vi "FlexDDS-NG_USB_ExampleJTedit.vi"() -> ()   [LabVIEW 2016]
uses:
  <vilib>/Utility/xml.llb/Read From XML File(string).vi
  <vilib>/Utility/xml.llb/Write to XML File(string).vi
panel:
  in  "Interactive on/off":T1(ring)
  out "return count":u32=6435
  in  "Store data":enum32{"Save settings", "Don't save settings"}(tab)=enum."Don't save settings"
  in  "XML File Path WRITE":path=path "U:/Dokumente/Bachelorarbeit/Labview/FlexDDS-NG/conf/settings_s_curve_up_down.xml"
  in  "Data source":T2(tab)=enum."Generate data with function"
  in  "XML File Path READ":path=path "U:/Dokumente/Bachelorarbeit/Labview/FlexDDS-NG/conf/settings_4consecutive_falling.xml"
  in  "Select curve form":enum32{"S curve", "Exp curve"}(tab)
  in  "s curve parameters":cluster{"k":dbl}={"k"=10.0}
  in  "exp curve parameters":cluster{"k":dbl}={"k"=5.0}
  in  "parameters non-constant channel":T3={"Number of steps"=40, "time [ms]"=10000.0, "start frequency [Hz]"=80000000.0, "end frequency [Hz]"=82000000.0}
  in  "constant frequency":dbl=80000000.0 format="%#_13g"
  in  "Constant Channel":T4(ring)
  in  "CFR2 bits":T5={"Enable ASF from STP (F)"=FALSE, "Digital ramp enable (F)"=TRUE, "Digital ramp no-dwell high (F)"=FALSE, "Digital ramp no-dwell low (F)"=FALSE, "Matched latency enable (T)"=TRUE, "Parallel data port enable (F)"=FALSE}
  in  "CFR1 bits":T6={"RAM enable (F)"=FALSE, "Manual OSK external control (F)"=FALSE, "Inverse sinc filter enable (T)"=TRUE, "DDS sine (/cosine) output (F)"=FALSE, "Load LRR at I/O update (F)"=FALSE, "Autoclear digital ramp accumulator (F)"=TRUE, "Autoclear phase accumulator (F)"=FALSE, "Clear digital ramp accumulator (F)"=FALSE, "Clear phase accumulator (F)"=FALSE, "Load ARR at I/O update (F)"=FALSE, "OSK enable (F)"=FALSE, "Select Auto OSK (F)"=FALSE}
  in  "Trigger before sequence of sweeps":T7(ring)
  out "appended instruction string 2":string="dds reset\rdcp spi:CFR1=0x404000\rdcp spi:CFR2=0x80080\rdcp 0 spi:STP0=0x3FFF0000028F5C29\rdcp 1 spi:STP0=0x3FFF0000028F5C29\rdcp 0 spi:DRL=0x147C0118147BC1DB\rdcp 0 spi:DRSS=0xFFFFFFFF00000003\rdcp 0 spi:DRR=0x2D3E\rdcp 0 update:u-d\rdcp 0 update:+d\rdcp 1 spi:DRL=0x147AE148147AE148\rdcp 1 spi:DRSS=0xFFFFFFFF00000000\rdcp 1 spi:DRR=0xFFFF\rdcp 1 update:u-d\rdcp 1 update:+d\rdcp wait:1h:\rdcp wait::DROVER\rdcp 0 spi:DRL=0x147C51F1147C0118\rdcp 0 spi:DRSS=0xFFFFFFFF00000004\rdcp 0 spi:DRR=0x2F2F\rdcp 0 update:u-d\rdcp 0 update:+d\rdcp wait:1h:\rdcp wait::DROVER\rdcp 0 spi:DRL=0x147CB92D147C51F1\rdcp 0 spi:DRSS=0xFFFFFFFF00000017\rdcp 0 spi:DRR=0xD478\rdcp 0 update:u-d\rdcp 0 update:+d\rdcp wait:1h:\rdcp wait::DROVER\rdcp 0 spi:DRL=0x147D3CCC147CB92D\rdcp 0 spi:DRSS=0xFFFFFFFF00000009\rdcp 0 spi:DRR=0x4136\rdcp 0 update:u-d\rdcp 0 update:+d\rdcp wait:1h:\rdcp wait::DROVER\rdcp 0 spi:DRL=0x147DE446147D3CCC\rdcp 0 spi:DRSS=0xFFFFFFFF0000000D\rdcp 0 spi:DRR=0x4A07\rdcp 0 update:u-d\rdcp 0 update:+d\rdcp wait:1h:\rdcp wait::DROVER\rdcp 0 spi:DRL=0x147EB8D6147DE446\rdcp 0 spi:DRSS=0xFFFFFFFF0000002B\rdcp 0 spi:DRR=0xC0EC\rdcp 0 update:u-d\rdcp 0 update:+d\rdcp wait:1h:\rdcp wait::DROVER\rdcp 0 spi:DRL=0x147FC5C3147EB8D6\rdcp 0 spi:DRSS=0xFFFFFFFF00000006\rdcp 0 spi:DRR=0x1547\rdcp 0 update:u-d\rdcp 0 update:+d\rdcp wait:1h:\rdcp wait::DROVER\rdcp 0 spi:DRL=0x148118A1147FC5C3\rdcp 0 spi:DRSS=0xFFFFFFFF0000001C\rdcp 0 spi:DRR=0x4ECD\rdcp 0 update:u-d\rdcp 0 update:+d\rdcp wait:1h:\rdcp wait::DROVER\rdcp 0 spi:DRL=0x1482C174148118A1\rdcp 0 spi:DRSS=0xFFFFFFFF00000049\rdcp 0 spi:DRR=0xA3E0\rdcp 0 update:u-d\rdcp 0 update:+d\rdcp wait:1h:\rdcp wait::DROVER\rdcp 0 spi:DRL=0x1484D2A81482C174\rdcp 0 spi:DRSS=0xFFFFFFFF00000003\rdcp 0 spi:DRR=0x568\rdcp 0 update:u-d\rdcp 0 update:+d\rdcp wait:1h:\rdcp wait::DROVER\rdcp 0 spi:DRL=0x148760AD1484D2A8\rdcp 0 spi:DRSS=0xFFFFFFFF0000008C\rdcp 0 spi:DRR=0xCC25\rdcp 0 update:u-d\rdcp 0 update:+d\rdcp wait:1h:\rdcp wait::DROVER\rdcp 0 spi:DRL=0x148A8111148760AD\rdcp 0 spi:DRSS=0xFFFFFFFF00000049\rdcp 0 spi:DRR=0x56FB\rdcp 0 update:u-d\rdcp 0 update:+d\rdcp wait:1h:\rdcp wait::DROVER\rdcp 0 spi:DRL=0x148E48EB148A8111\rdcp 0 spi:DRSS=0xFFFFFFFF00000004\rdcp 0 spi:DRR=0x3F1\rdcp 0 update:u-d\rdcp 0 update:+d\rdcp wait:1h:\rdcp wait::DROVER\rdcp 0 spi:DRL=0x1492CA77148E48EB\rdcp 0 spi:DRSS=0xFFFFFFFF000000A0\rdcp 0 spi:DRR=0x8447\rdcp 0 update:u-d\rdcp 0 update:+d\rdcp wait:1h:\rdcp wait::DROVER\rdcp 0 spi:DRL=0x149811DB1492CA77\rdcp 0 spi:DRSS=0xFFFFFFFF000000D0\rdcp 0 spi:DRR=0x92C9\rdcp 0 update:u-d\rdcp 0 update:+d\rdcp wait:1h:\rdcp wait::DROVER\rdcp 0 spi:DRL=0x149E2175149811DB\rdcp 0 spi:DRSS=0xFFFFFFFF00000100\rdcp 0 spi:DRR=0x9D59\rdcp 0 update:u-d\rdcp 0 update:+d\rdcp wait:1h:\rdcp wait::DROVER\rdcp 0 spi:DRL=0x14A4EE42149E2175\rdcp 0 spi:DRSS=0xFFFFFFFF000000C7\rdcp 0 spi:DRR=0x6D05\rdcp 0 update:u-d\rdcp 0 update:+d\rdcp wait:1h:\rdcp wait::DROVER\rdcp 0 spi:DRL=0x14AC5D7114A4EE42\rdcp 0 spi:DRSS=0xFFFFFFFF00000019\rdcp 0 spi:DRR=0xC87\rdcp 0 update:u-d\rdcp 0 update:+d\rdcp wait:1h:\rdcp wait::DROVER\rdcp 0 spi:DRL=0x14B4443314AC5D71\rdcp 0 spi:DRSS=0xFFFFFFFF00000021\rdcp 0 spi:DRR=0xF8F\rdcp 0 update:u-d\rdcp 0 update:+d\rdcp wait:1h:\rdcp wait::DROVER\rdcp 0 spi:DRL=0x14BC6A7F14B44433\rdcp 0 spi:DRSS=0xFFFFFFFF0000014D\rdcp 0 spi:DRR=0x9838\rdcp 0 update:u-d\rdcp 0 update:+d\rdcp wait:1h:\rdcp wait::DROVER\rdcp 0 spi:DRL=0x14C490CB14BC6A7F\rdcp 0 spi:DRSS=0xFFFFFFFF0000014D\rdcp 0 spi:DRR=0x9838\rdcp 0 update:u-d\rdcp 0 update:+d\rdcp wait:1h:\rdcp wait::DROVER\rdcp 0 spi:DRL=0x14CC778D14C490CB\rdcp 0 spi:DRSS=0xFFFFFFFF00000021\rdcp 0 spi:DRR=0xF8F\rdcp 0 update:u-d\rdcp 0 update:+d\rdcp wait:1h:\rdcp wait::DROVER\rdcp 0 spi:DRL=0x14D3E6BC14CC778D\rdcp 0 spi:DRSS=0xFFFFFFFF00000019\rdcp 0 spi:DRR=0xC87\rdcp 0 update:u-d\rdcp 0 update:+d\rdcp wait:1h:\rdcp wait::DROVER\rdcp 0 spi:DRL=0x14DAB38914D3E6BC\rdcp 0 spi:DRSS=0xFFFFFFFF000000C7\rdcp 0 spi:DRR=0x6D05\rdcp 0 update:u-d\rdcp 0 update:+d\rdcp wait:1h:\rdcp wait::DROVER\rdcp 0 spi:DRL=0x14E0C32314DAB389\rdcp 0 spi:DRSS=0xFFFFFFFF00000100\rdcp 0 spi:DRR=0x9D59\rdcp 0 update:u-d\rdcp 0 update:+d\rdcp wait:1h:\rdcp wait::DROVER\rdcp 0 spi:DRL=0x14E60A8714E0C323\rdcp 0 spi:DRSS=0xFFFFFFFF000000D0\rdcp 0 spi:DRR=0x92C9\rdcp 0 update:u-d\rdcp 0 update:+d\rdcp wait:1h:\rdcp wait::DROVER\rdcp 0 spi:DRL=0x14EA8C1314E60A87\rdcp 0 spi:DRSS=0xFFFFFFFF000000A0\rdcp 0 spi:DRR=0x8447\rdcp 0 update:u-d\rdcp 0 update:+d\rdcp wait:1h:\rdcp wait::DROVER\rdcp 0 spi:DRL=0x14EE53ED14EA8C13\rdcp 0 spi:DRSS=0xFFFFFFFF00000004\rdcp 0 spi:DRR=0x3F1\rdcp 0 update:u-d\rdcp 0 update:+d\rdcp wait:1h:\rdcp wait::DROVER\rdcp 0 spi:DRL=0x14F1745114EE53ED\rdcp 0 spi:DRSS=0xFFFFFFFF00000049\rdcp 0 spi:DRR=0x56FB\rdcp 0 update:u-d\rdcp 0 update:+d\rdcp wait:1h:\rdcp wait::DROVER\rdcp 0 spi:DRL=0x14F4025514F17451\rdcp 0 spi:DRSS=0xFFFFFFFF0000008C\rdcp 0 spi:DRR=0xCC25\rdcp 0 update:u-d\rdcp 0 update:+d\rdcp wait:1h:\rdcp wait::DROVER\rdcp 0 spi:DRL=0x14F6138A14F40255\rdcp 0 spi:DRSS=0xFFFFFFFF00000003\rdcp 0 spi:DRR=0x568\rdcp 0 update:u-d\rdcp 0 update:+d\rdcp wait:1h:\rdcp wait::DROVER\rdcp 0 spi:DRL=0x14F7BC5D14F6138A\rdcp 0 spi:DRSS=0xFFFFFFFF00000049\rdcp 0 spi:DRR=0xA3E0\rdcp 0 update:u-d\rdcp 0 update:+d\rdcp wait:1h:\rdcp wait::DROVER\rdcp 0 spi:DRL=0x14F90F3B14F7BC5D\rdcp 0 spi:DRSS=0xFFFFFFFF0000001C\rdcp 0 spi:DRR=0x4ECD\rdcp 0 update:u-d\rdcp 0 update:+d\rdcp wait:1h:\rdcp wait::DROVER\rdcp 0 spi:DRL=0x14FA1C2814F90F3B\rdcp 0 spi:DRSS=0xFFFFFFFF00000006\rdcp 0 spi:DRR=0x1547\rdcp 0 update:u-d\rdcp 0 update:+d\rdcp wait:1h:\rdcp wait::DROVER\rdcp 0 spi:DRL=0x14FAF0B814FA1C28\rdcp 0 spi:DRSS=0xFFFFFFFF0000002B\rdcp 0 spi:DRR=0xC0EC\rdcp 0 update:u-d\rdcp 0 update:+d\rdcp wait:1h:\rdcp wait::DROVER\rdcp 0 spi:DRL=0x14FB983214FAF0B8\rdcp 0 spi:DRSS=0xFFFFFFFF0000000D\rdcp 0 spi:DRR=0x4A07\rdcp 0 update:u-d\rdcp 0 update:+d\rdcp wait:1h:\rdcp wait::DROVER\rdcp 0 spi:DRL=0x14FC1BD114FB9832\rdcp 0 spi:DRSS=0xFFFFFFFF00000009\rdcp 0 spi:DRR=0x4136\rdcp 0 update:u-d\rdcp 0 update:+d\rdcp wait:1h:\rdcp wait::DROVER\rdcp 0 spi:DRL=0x14FC830D14FC1BD1\rdcp 0 spi:DRSS=0xFFFFFFFF00000017\rdcp 0 spi:DRR=0xD478\rdcp 0 update:u-d\rdcp 0 update:+d\rdcp wait:1h:\rdcp wait::DROVER\rdcp 0 spi:DRL=0x14FCD3E614FC830D\rdcp 0 spi:DRSS=0xFFFFFFFF00000004\rdcp 0 spi:DRR=0x2F2F\rdcp 0 update:u-d\rdcp 0 update:+d\rdcp wait:1h:\rdcp wait::DROVER\rdcp 0 spi:DRL=0x14FD132314FCD3E6\rdcp 0 spi:DRSS=0xFFFFFFFF00000003\rdcp 0 spi:DRR=0x2D3E\rdcp 0 update:u-d\rdcp 0 update:+d\rdcp wait:1h:\rdcp wait::DROVER\rdcp 0 spi:DRL=0x14FD448E14FD1323\rdcp 0 spi:DRSS=0xFFFFFFFF00000002\rdcp 0 spi:DRR=0x2699\rdcp 0 update:u-d\rdcp 0 update:+d\rdcp wait:1h:\rdcp wait::DROVER\rdcp start\r"
  out "frequency-time plot":T8(graph)=[{[{"total time[ms]"=0.0, "f1 [Hz] CH0"=80013385.70184857}, {"total time[ms]"=250.0, "f1 [Hz] CH0"=80017154.97082743}, {"total time[ms]"=250.0, "f1 [Hz] CH0"=80017154.97082743}, {"total time[ms]"=500.0, "f1 [Hz] CH0"=80021973.8852612}, {"total time[ms]"=500.0, "f1 [Hz] CH0"=80021973.8852612}, {"total time[ms]"=750.0, "f1 [Hz] CH0"=80028127.2540865}, {"total time[ms]"=750.0, "f1 [Hz] CH0"=80028127.2540865}, {"total time[ms]"=1000.0, "f1 [Hz] CH0"=80035972.41992418}, {"total time[ms]"=1000.0, "f1 [Hz] CH0"=80035972.41992418}, {"total time[ms]"=1250.0, "f1 [Hz] CH0"=80045954.73982005}, {"total time[ms]"=1250.0, "f1 [Hz] CH0"=80045954.73982005}, {"total time[ms]"=1500.0, "f1 [Hz] CH0"=80058624.46150272}, {"total time[ms]"=1500.0, "f1 [Hz] CH0"=80058624.46150272}, {"total time[ms]"=1750.0, "f1 [Hz] CH0"=80074653.77468826}, {"total time[ms]"=1750.0, "f1 [Hz] CH0"=80074653.77468826}, {"total time[ms]"=2000.0, "f1 [Hz] CH0"=80094851.74635513}, {"total time[ms]"=2000.0, "f1 [Hz] CH0"=80094851.74635513}, {"total time[ms]"=2250.0, "f1 [Hz] CH0"=80120173.30034801}, {"total time[ms]"=2250.0, "f1 [Hz] CH0"=80120173.30034801}, {"total time[ms]"=2500.0, "f1 [Hz] CH0"=80151716.36004248}, {"total time[ms]"=2500.0, "f1 [Hz] CH0"=80151716.36004248}, {"total time[ms]"=2750.0, "f1 [Hz] CH0"=80190698.92979822}, {"total time[ms]"=2750.0, "f1 [Hz] CH0"=80190698.92979822}, {"total time[ms]"=3000.0, "f1 [Hz] CH0"=80238405.84404424}, {"total time[ms]"=3000.0, "f1 [Hz] CH0"=80238405.84404424}, {"total time[ms]"=3250.0, "f1 [Hz] CH0"=80296094.39606337}, {"total time[ms]"=3250.0, "f1 [Hz] CH0"=80296094.39606337}, {"total time[ms]"=3500.0, "f1 [Hz] CH0"=80364851.04761271}, {"total time[ms]"=3500.0, "f1 [Hz] CH0"=80364851.04761271}, {"total time[ms]"=3750.0, "f1 [Hz] CH0"=80445400.27765062}, {"total time[ms]"=3750.0, "f1 [Hz] CH0"=80445400.27765062}, {"total time[ms]"=4000.0, "f1 [Hz] CH0"=80537882.84273998}, {"total time[ms]"=4000.0, "f1 [Hz] CH0"=80537882.84273998}, {"total time[ms]"=4250.0, "f1 [Hz] CH0"=80641642.60164921}, {"total time[ms]"=4250.0, "f1 [Hz] CH0"=80641642.60164921}, {"total time[ms]"=4500.0, "f1 [Hz] CH0"=80755081.3375963}, {"total time[ms]"=4500.0, "f1 [Hz] CH0"=80755081.3375963}, {"total time[ms]"=4750.0, "f1 [Hz] CH0"=80875646.9982284}, {"total time[ms]"=4750.0, "f1 [Hz] CH0"=80875646.9982284}, {"total time[ms]"=5000.0, "f1 [Hz] CH0"=81000000.0}, {"total time[ms]"=5000.0, "f1 [Hz] CH0"=81000000.0}, {"total time[ms]"=5250.0, "f1 [Hz] CH0"=81124353.0017716}, {"total time[ms]"=5250.0, "f1 [Hz] CH0"=81124353.0017716}, {"total time[ms]"=5500.0, "f1 [Hz] CH0"=81244918.6624037}, {"total time[ms]"=5500.0, "f1 [Hz] CH0"=81244918.6624037}, {"total time[ms]"=5750.0, "f1 [Hz] CH0"=81358357.39835079}, {"total time[ms]"=5750.0, "f1 [Hz] CH0"=81358357.39835079}, {"total time[ms]"=6000.0, "f1 [Hz] CH0"=81462117.15726002}, {"total time[ms]"=6000.0, "f1 [Hz] CH0"=81462117.15726002}, {"total time[ms]"=6250.0, "f1 [Hz] CH0"=81554599.72234938}, {"total time[ms]"=6250.0, "f1 [Hz] CH0"=81554599.72234938}, {"total time[ms]"=6500.0, "f1 [Hz] CH0"=81635148.95238729}, {"total time[ms]"=6500.0, "f1 [Hz] CH0"=81635148.95238729}, {"total time[ms]"=6750.0, "f1 [Hz] CH0"=81703905.60393663}, {"total time[ms]"=6750.0, "f1 [Hz] CH0"=81703905.60393663}, {"total time[ms]"=7000.0, "f1 [Hz] CH0"=81761594.15595576}, {"total time[ms]"=7000.0, "f1 [Hz] CH0"=81761594.15595576}, {"total time[ms]"=7250.0, "f1 [Hz] CH0"=81809301.07020178}, {"total time[ms]"=7250.0, "f1 [Hz] CH0"=81809301.07020178}, {"total time[ms]"=7500.0, "f1 [Hz] CH0"=81848283.63995752}, {"total time[ms]"=7500.0, "f1 [Hz] CH0"=81848283.63995752}, {"total time[ms]"=7750.0, "f1 [Hz] CH0"=81879826.69965199}, {"total time[ms]"=7750.0, "f1 [Hz] CH0"=81879826.69965199}, {"total time[ms]"=8000.0, "f1 [Hz] CH0"=81905148.25364487}, {"total time[ms]"=8000.0, "f1 [Hz] CH0"=81905148.25364487}, {"total time[ms]"=8250.0, "f1 [Hz] CH0"=81925346.22531174}, {"total time[ms]"=8250.0, "f1 [Hz] CH0"=81925346.22531174}, {"total time[ms]"=8500.0, "f1 [Hz] CH0"=81941375.53849728}, {"total time[ms]"=8500.0, "f1 [Hz] CH0"=81941375.53849728}, {"total time[ms]"=8750.0, "f1 [Hz] CH0"=81954045.26017995}, {"total time[ms]"=8750.0, "f1 [Hz] CH0"=81954045.26017995}, {"total time[ms]"=9000.0, "f1 [Hz] CH0"=81964027.58007582}, {"total time[ms]"=9000.0, "f1 [Hz] CH0"=81964027.58007582}, {"total time[ms]"=9250.0, "f1 [Hz] CH0"=81971872.7459135}, {"total time[ms]"=9250.0, "f1 [Hz] CH0"=81971872.7459135}, {"total time[ms]"=9500.0, "f1 [Hz] CH0"=81978026.1147388}, {"total time[ms]"=9500.0, "f1 [Hz] CH0"=81978026.1147388}, {"total time[ms]"=9750.0, "f1 [Hz] CH0"=81982845.02917257}, {"total time[ms]"=9750.0, "f1 [Hz] CH0"=81982845.02917257}, {"total time[ms]"=10000.0, "f1 [Hz] CH0"=81986614.29815143}, {"total time[ms]"=10000.0, "f1 [Hz] CH0"=81986614.29815143}, {"total time[ms]"=10250.0, "f1 [Hz] CH0"=81989559.74861288}]}, {[{"total time[ms]"=0.0, "f1 [Hz] CH0"=80000000.0}, {"total time[ms]"=250.0, "f1 [Hz] CH0"=80000000.0}, {"total time[ms]"=250.0, "f1 [Hz] CH0"=80000000.0}, {"total time[ms]"=500.0, "f1 [Hz] CH0"=80000000.0}, {"total time[ms]"=500.0, "f1 [Hz] CH0"=80000000.0}, {"total time[ms]"=750.0, "f1 [Hz] CH0"=80000000.0}, {"total time[ms]"=750.0, "f1 [Hz] CH0"=80000000.0}, {"total time[ms]"=1000.0, "f1 [Hz] CH0"=80000000.0}, {"total time[ms]"=1000.0, "f1 [Hz] CH0"=80000000.0}, {"total time[ms]"=1250.0, "f1 [Hz] CH0"=80000000.0}, {"total time[ms]"=1250.0, "f1 [Hz] CH0"=80000000.0}, {"total time[ms]"=1500.0, "f1 [Hz] CH0"=80000000.0}, {"total time[ms]"=1500.0, "f1 [Hz] CH0"=80000000.0}, {"total time[ms]"=1750.0, "f1 [Hz] CH0"=80000000.0}, {"total time[ms]"=1750.0, "f1 [Hz] CH0"=80000000.0}, {"total time[ms]"=2000.0, "f1 [Hz] CH0"=80000000.0}, {"total time[ms]"=2000.0, "f1 [Hz] CH0"=80000000.0}, {"total time[ms]"=2250.0, "f1 [Hz] CH0"=80000000.0}, {"total time[ms]"=2250.0, "f1 [Hz] CH0"=80000000.0}, {"total time[ms]"=2500.0, "f1 [Hz] CH0"=80000000.0}, {"total time[ms]"=2500.0, "f1 [Hz] CH0"=80000000.0}, {"total time[ms]"=2750.0, "f1 [Hz] CH0"=80000000.0}, {"total time[ms]"=2750.0, "f1 [Hz] CH0"=80000000.0}, {"total time[ms]"=3000.0, "f1 [Hz] CH0"=80000000.0}, {"total time[ms]"=3000.0, "f1 [Hz] CH0"=80000000.0}, {"total time[ms]"=3250.0, "f1 [Hz] CH0"=80000000.0}, {"total time[ms]"=3250.0, "f1 [Hz] CH0"=80000000.0}, {"total time[ms]"=3500.0, "f1 [Hz] CH0"=80000000.0}, {"total time[ms]"=3500.0, "f1 [Hz] CH0"=80000000.0}, {"total time[ms]"=3750.0, "f1 [Hz] CH0"=80000000.0}, {"total time[ms]"=3750.0, "f1 [Hz] CH0"=80000000.0}, {"total time[ms]"=4000.0, "f1 [Hz] CH0"=80000000.0}, {"total time[ms]"=4000.0, "f1 [Hz] CH0"=80000000.0}, {"total time[ms]"=4250.0, "f1 [Hz] CH0"=80000000.0}, {"total time[ms]"=4250.0, "f1 [Hz] CH0"=80000000.0}, {"total time[ms]"=4500.0, "f1 [Hz] CH0"=80000000.0}, {"total time[ms]"=4500.0, "f1 [Hz] CH0"=80000000.0}, {"total time[ms]"=4750.0, "f1 [Hz] CH0"=80000000.0}, {"total time[ms]"=4750.0, "f1 [Hz] CH0"=80000000.0}, {"total time[ms]"=5000.0, "f1 [Hz] CH0"=80000000.0}, {"total time[ms]"=5000.0, "f1 [Hz] CH0"=80000000.0}, {"total time[ms]"=5250.0, "f1 [Hz] CH0"=80000000.0}, {"total time[ms]"=5250.0, "f1 [Hz] CH0"=80000000.0}, {"total time[ms]"=5500.0, "f1 [Hz] CH0"=80000000.0}, {"total time[ms]"=5500.0, "f1 [Hz] CH0"=80000000.0}, {"total time[ms]"=5750.0, "f1 [Hz] CH0"=80000000.0}, {"total time[ms]"=5750.0, "f1 [Hz] CH0"=80000000.0}, {"total time[ms]"=6000.0, "f1 [Hz] CH0"=80000000.0}, {"total time[ms]"=6000.0, "f1 [Hz] CH0"=80000000.0}, {"total time[ms]"=6250.0, "f1 [Hz] CH0"=80000000.0}, {"total time[ms]"=6250.0, "f1 [Hz] CH0"=80000000.0}, {"total time[ms]"=6500.0, "f1 [Hz] CH0"=80000000.0}, {"total time[ms]"=6500.0, "f1 [Hz] CH0"=80000000.0}, {"total time[ms]"=6750.0, "f1 [Hz] CH0"=80000000.0}, {"total time[ms]"=6750.0, "f1 [Hz] CH0"=80000000.0}, {"total time[ms]"=7000.0, "f1 [Hz] CH0"=80000000.0}, {"total time[ms]"=7000.0, "f1 [Hz] CH0"=80000000.0}, {"total time[ms]"=7250.0, "f1 [Hz] CH0"=80000000.0}, {"total time[ms]"=7250.0, "f1 [Hz] CH0"=80000000.0}, {"total time[ms]"=7500.0, "f1 [Hz] CH0"=80000000.0}, {"total time[ms]"=7500.0, "f1 [Hz] CH0"=80000000.0}, {"total time[ms]"=7750.0, "f1 [Hz] CH0"=80000000.0}, {"total time[ms]"=7750.0, "f1 [Hz] CH0"=80000000.0}, {"total time[ms]"=8000.0, "f1 [Hz] CH0"=80000000.0}, {"total time[ms]"=8000.0, "f1 [Hz] CH0"=80000000.0}, {"total time[ms]"=8250.0, "f1 [Hz] CH0"=80000000.0}, {"total time[ms]"=8250.0, "f1 [Hz] CH0"=80000000.0}, {"total time[ms]"=8500.0, "f1 [Hz] CH0"=80000000.0}, {"total time[ms]"=8500.0, "f1 [Hz] CH0"=80000000.0}, {"total time[ms]"=8750.0, "f1 [Hz] CH0"=80000000.0}, {"total time[ms]"=8750.0, "f1 [Hz] CH0"=80000000.0}, {"total time[ms]"=9000.0, "f1 [Hz] CH0"=80000000.0}, {"total time[ms]"=9000.0, "f1 [Hz] CH0"=80000000.0}, {"total time[ms]"=9250.0, "f1 [Hz] CH0"=80000000.0}, {"total time[ms]"=9250.0, "f1 [Hz] CH0"=80000000.0}, {"total time[ms]"=9500.0, "f1 [Hz] CH0"=80000000.0}, {"total time[ms]"=9500.0, "f1 [Hz] CH0"=80000000.0}, {"total time[ms]"=9750.0, "f1 [Hz] CH0"=80000000.0}, {"total time[ms]"=9750.0, "f1 [Hz] CH0"=80000000.0}, {"total time[ms]"=10000.0, "f1 [Hz] CH0"=80000000.0}, {"total time[ms]"=10000.0, "f1 [Hz] CH0"=80000000.0}, {"total time[ms]"=10250.0, "f1 [Hz] CH0"=80000000.0}]}]
  in  "Control Elements Array":T9(array[cluster])=[{"STEP"=0, "time[ms]"=250.0, "time tolerance[us]"=0.01, "CH0"=TRUE, "rel. amplitude CH0"=1.0, "phase [°] CH0"=0.0, "f0 [Hz] CH0"=80013385.70184857, "f1 [Hz] CH0"=80017154.97082743, "CH1"=TRUE, "rel. amplitude CH1"=1.0, "phase [°] CH1"=0.0, "f0 [Hz] CH1"=80000000.0, "f1 [Hz] CH1"=80000000.0}, {"STEP"=0, "time[ms]"=250.0, "time tolerance[us]"=0.01, "CH0"=TRUE, "rel. amplitude CH0"=1.0, "phase [°] CH0"=0.0, "f0 [Hz] CH0"=80017154.97082743, "f1 [Hz] CH0"=80021973.8852612, "CH1"=FALSE, "rel. amplitude CH1"=1.0, "phase [°] CH1"=0.0, "f0 [Hz] CH1"=80000000.0, "f1 [Hz] CH1"=80000000.0}, {"STEP"=0, "time[ms]"=250.0, "time tolerance[us]"=0.01, "CH0"=TRUE, "rel. amplitude CH0"=1.0, "phase [°] CH0"=0.0, "f0 [Hz] CH0"=80021973.8852612, "f1 [Hz] CH0"=80028127.2540865, "CH1"=FALSE, "rel. amplitude CH1"=1.0, "phase [°] CH1"=0.0, "f0 [Hz] CH1"=80000000.0, "f1 [Hz] CH1"=80000000.0}, {"STEP"=0, "time[ms]"=250.0, "time tolerance[us]"=0.01, "CH0"=TRUE, "rel. amplitude CH0"=1.0, "phase [°] CH0"=0.0, "f0 [Hz] CH0"=80028127.2540865, "f1 [Hz] CH0"=80035972.41992418, "CH1"=FALSE, "rel. amplitude CH1"=1.0, "phase [°] CH1"=0.0, "f0 [Hz] CH1"=80000000.0, "f1 [Hz] CH1"=80000000.0}, {"STEP"=0, "time[ms]"=250.0, "time tolerance[us]"=0.01, "CH0"=TRUE, "rel. amplitude CH0"=1.0, "phase [°] CH0"=0.0, "f0 [Hz] CH0"=80035972.41992418, "f1 [Hz] CH0"=80045954.73982005, "CH1"=FALSE, "rel. amplitude CH1"=1.0, "phase [°] CH1"=0.0, "f0 [Hz] CH1"=80000000.0, "f1 [Hz] CH1"=80000000.0}, {"STEP"=0, "time[ms]"=250.0, "time tolerance[us]"=0.01, "CH0"=TRUE, "rel. amplitude CH0"=1.0, "phase [°] CH0"=0.0, "f0 [Hz] CH0"=80045954.73982005, "f1 [Hz] CH0"=80058624.46150272, "CH1"=FALSE, "rel. amplitude CH1"=1.0, "phase [°] CH1"=0.0, "f0 [Hz] CH1"=80000000.0, "f1 [Hz] CH1"=80000000.0}, {"STEP"=0, "time[ms]"=250.0, "time tolerance[us]"=0.01, "CH0"=TRUE, "rel. amplitude CH0"=1.0, "phase [°] CH0"=0.0, "f0 [Hz] CH0"=80058624.46150272, "f1 [Hz] CH0"=80074653.77468826, "CH1"=FALSE, "rel. amplitude CH1"=1.0, "phase [°] CH1"=0.0, "f0 [Hz] CH1"=80000000.0, "f1 [Hz] CH1"=80000000.0}, {"STEP"=0, "time[ms]"=250.0, "time tolerance[us]"=0.01, "CH0"=TRUE, "rel. amplitude CH0"=1.0, "phase [°] CH0"=0.0, "f0 [Hz] CH0"=80074653.77468826, "f1 [Hz] CH0"=80094851.74635513, "CH1"=FALSE, "rel. amplitude CH1"=1.0, "phase [°] CH1"=0.0, "f0 [Hz] CH1"=80000000.0, "f1 [Hz] CH1"=80000000.0}, {"STEP"=0, "time[ms]"=250.0, "time tolerance[us]"=0.01, "CH0"=TRUE, "rel. amplitude CH0"=1.0, "phase [°] CH0"=0.0, "f0 [Hz] CH0"=80094851.74635513, "f1 [Hz] CH0"=80120173.30034801, "CH1"=FALSE, "rel. amplitude CH1"=1.0, "phase [°] CH1"=0.0, "f0 [Hz] CH1"=80000000.0, "f1 [Hz] CH1"=80000000.0}, {"STEP"=0, "time[ms]"=250.0, "time tolerance[us]"=0.01, "CH0"=TRUE, "rel. amplitude CH0"=1.0, "phase [°] CH0"=0.0, "f0 [Hz] CH0"=80120173.30034801, "f1 [Hz] CH0"=80151716.36004248, "CH1"=FALSE, "rel. amplitude CH1"=1.0, "phase [°] CH1"=0.0, "f0 [Hz] CH1"=80000000.0, "f1 [Hz] CH1"=80000000.0}, {"STEP"=0, "time[ms]"=250.0, "time tolerance[us]"=0.01, "CH0"=TRUE, "rel. amplitude CH0"=1.0, "phase [°] CH0"=0.0, "f0 [Hz] CH0"=80151716.36004248, "f1 [Hz] CH0"=80190698.92979822, "CH1"=FALSE, "rel. amplitude CH1"=1.0, "phase [°] CH1"=0.0, "f0 [Hz] CH1"=80000000.0, "f1 [Hz] CH1"=80000000.0}, {"STEP"=0, "time[ms]"=250.0, "time tolerance[us]"=0.01, "CH0"=TRUE, "rel. amplitude CH0"=1.0, "phase [°] CH0"=0.0, "f0 [Hz] CH0"=80190698.92979822, "f1 [Hz] CH0"=80238405.84404424, "CH1"=FALSE, "rel. amplitude CH1"=1.0, "phase [°] CH1"=0.0, "f0 [Hz] CH1"=80000000.0, "f1 [Hz] CH1"=80000000.0}, {"STEP"=0, "time[ms]"=250.0, "time tolerance[us]"=0.01, "CH0"=TRUE, "rel. amplitude CH0"=1.0, "phase [°] CH0"=0.0, "f0 [Hz] CH0"=80238405.84404424, "f1 [Hz] CH0"=80296094.39606337, "CH1"=FALSE, "rel. amplitude CH1"=1.0, "phase [°] CH1"=0.0, "f0 [Hz] CH1"=80000000.0, "f1 [Hz] CH1"=80000000.0}, {"STEP"=0, "time[ms]"=250.0, "time tolerance[us]"=0.01, "CH0"=TRUE, "rel. amplitude CH0"=1.0, "phase [°] CH0"=0.0, "f0 [Hz] CH0"=80296094.39606337, "f1 [Hz] CH0"=80364851.04761271, "CH1"=FALSE, "rel. amplitude CH1"=1.0, "phase [°] CH1"=0.0, "f0 [Hz] CH1"=80000000.0, "f1 [Hz] CH1"=80000000.0}, {"STEP"=0, "time[ms]"=250.0, "time tolerance[us]"=0.01, "CH0"=TRUE, "rel. amplitude CH0"=1.0, "phase [°] CH0"=0.0, "f0 [Hz] CH0"=80364851.04761271, "f1 [Hz] CH0"=80445400.27765062, "CH1"=FALSE, "rel. amplitude CH1"=1.0, "phase [°] CH1"=0.0, "f0 [Hz] CH1"=80000000.0, "f1 [Hz] CH1"=80000000.0}, {"STEP"=0, "time[ms]"=250.0, "time tolerance[us]"=0.01, "CH0"=TRUE, "rel. amplitude CH0"=1.0, "phase [°] CH0"=0.0, "f0 [Hz] CH0"=80445400.27765062, "f1 [Hz] CH0"=80537882.84273998, "CH1"=FALSE, "rel. amplitude CH1"=1.0, "phase [°] CH1"=0.0, "f0 [Hz] CH1"=80000000.0, "f1 [Hz] CH1"=80000000.0}, {"STEP"=0, "time[ms]"=250.0, "time tolerance[us]"=0.01, "CH0"=TRUE, "rel. amplitude CH0"=1.0, "phase [°] CH0"=0.0, "f0 [Hz] CH0"=80537882.84273998, "f1 [Hz] CH0"=80641642.60164921, "CH1"=FALSE, "rel. amplitude CH1"=1.0, "phase [°] CH1"=0.0, "f0 [Hz] CH1"=80000000.0, "f1 [Hz] CH1"=80000000.0}, {"STEP"=0, "time[ms]"=250.0, "time tolerance[us]"=0.01, "CH0"=TRUE, "rel. amplitude CH0"=1.0, "phase [°] CH0"=0.0, "f0 [Hz] CH0"=80641642.60164921, "f1 [Hz] CH0"=80755081.3375963, "CH1"=FALSE, "rel. amplitude CH1"=1.0, "phase [°] CH1"=0.0, "f0 [Hz] CH1"=80000000.0, "f1 [Hz] CH1"=80000000.0}, {"STEP"=0, "time[ms]"=250.0, "time tolerance[us]"=0.01, "CH0"=TRUE, "rel. amplitude CH0"=1.0, "phase [°] CH0"=0.0, "f0 [Hz] CH0"=80755081.3375963, "f1 [Hz] CH0"=80875646.9982284, "CH1"=FALSE, "rel. amplitude CH1"=1.0, "phase [°] CH1"=0.0, "f0 [Hz] CH1"=80000000.0, "f1 [Hz] CH1"=80000000.0}, {"STEP"=0, "time[ms]"=250.0, "time tolerance[us]"=0.01, "CH0"=TRUE, "rel. amplitude CH0"=1.0, "phase [°] CH0"=0.0, "f0 [Hz] CH0"=80875646.9982284, "f1 [Hz] CH0"=81000000.0, "CH1"=FALSE, "rel. amplitude CH1"=1.0, "phase [°] CH1"=0.0, "f0 [Hz] CH1"=80000000.0, "f1 [Hz] CH1"=80000000.0}, {"STEP"=0, "time[ms]"=250.0, "time tolerance[us]"=0.01, "CH0"=TRUE, "rel. amplitude CH0"=1.0, "phase [°] CH0"=0.0, "f0 [Hz] CH0"=81000000.0, "f1 [Hz] CH0"=81124353.0017716, "CH1"=FALSE, "rel. amplitude CH1"=1.0, "phase [°] CH1"=0.0, "f0 [Hz] CH1"=80000000.0, "f1 [Hz] CH1"=80000000.0}, {"STEP"=0, "time[ms]"=250.0, "time tolerance[us]"=0.01, "CH0"=TRUE, "rel. amplitude CH0"=1.0, "phase [°] CH0"=0.0, "f0 [Hz] CH0"=81124353.0017716, "f1 [Hz] CH0"=81244918.6624037, "CH1"=FALSE, "rel. amplitude CH1"=1.0, "phase [°] CH1"=0.0, "f0 [Hz] CH1"=80000000.0, "f1 [Hz] CH1"=80000000.0}, {"STEP"=0, "time[ms]"=250.0, "time tolerance[us]"=0.01, "CH0"=TRUE, "rel. amplitude CH0"=1.0, "phase [°] CH0"=0.0, "f0 [Hz] CH0"=81244918.6624037, "f1 [Hz] CH0"=81358357.39835079, "CH1"=FALSE, "rel. amplitude CH1"=1.0, "phase [°] CH1"=0.0, "f0 [Hz] CH1"=80000000.0, "f1 [Hz] CH1"=80000000.0}, {"STEP"=0, "time[ms]"=250.0, "time tolerance[us]"=0.01, "CH0"=TRUE, "rel. amplitude CH0"=1.0, "phase [°] CH0"=0.0, "f0 [Hz] CH0"=81358357.39835079, "f1 [Hz] CH0"=81462117.15726002, "CH1"=FALSE, "rel. amplitude CH1"=1.0, "phase [°] CH1"=0.0, "f0 [Hz] CH1"=80000000.0, "f1 [Hz] CH1"=80000000.0}, {"STEP"=0, "time[ms]"=250.0, "time tolerance[us]"=0.01, "CH0"=TRUE, "rel. amplitude CH0"=1.0, "phase [°] CH0"=0.0, "f0 [Hz] CH0"=81462117.15726002, "f1 [Hz] CH0"=81554599.72234938, "CH1"=FALSE, "rel. amplitude CH1"=1.0, "phase [°] CH1"=0.0, "f0 [Hz] CH1"=80000000.0, "f1 [Hz] CH1"=80000000.0}, {"STEP"=0, "time[ms]"=250.0, "time tolerance[us]"=0.01, "CH0"=TRUE, "rel. amplitude CH0"=1.0, "phase [°] CH0"=0.0, "f0 [Hz] CH0"=81554599.72234938, "f1 [Hz] CH0"=81635148.95238729, "CH1"=FALSE, "rel. amplitude CH1"=1.0, "phase [°] CH1"=0.0, "f0 [Hz] CH1"=80000000.0, "f1 [Hz] CH1"=80000000.0}, {"STEP"=0, "time[ms]"=250.0, "time tolerance[us]"=0.01, "CH0"=TRUE, "rel. amplitude CH0"=1.0, "phase [°] CH0"=0.0, "f0 [Hz] CH0"=81635148.95238729, "f1 [Hz] CH0"=81703905.60393663, "CH1"=FALSE, "rel. amplitude CH1"=1.0, "phase [°] CH1"=0.0, "f0 [Hz] CH1"=80000000.0, "f1 [Hz] CH1"=80000000.0}, {"STEP"=0, "time[ms]"=250.0, "time tolerance[us]"=0.01, "CH0"=TRUE, "rel. amplitude CH0"=1.0, "phase [°] CH0"=0.0, "f0 [Hz] CH0"=81703905.60393663, "f1 [Hz] CH0"=81761594.15595576, "CH1"=FALSE, "rel. amplitude CH1"=1.0, "phase [°] CH1"=0.0, "f0 [Hz] CH1"=80000000.0, "f1 [Hz] CH1"=80000000.0}, {"STEP"=0, "time[ms]"=250.0, "time tolerance[us]"=0.01, "CH0"=TRUE, "rel. amplitude CH0"=1.0, "phase [°] CH0"=0.0, "f0 [Hz] CH0"=81761594.15595576, "f1 [Hz] CH0"=81809301.07020178, "CH1"=FALSE, "rel. amplitude CH1"=1.0, "phase [°] CH1"=0.0, "f0 [Hz] CH1"=80000000.0, "f1 [Hz] CH1"=80000000.0}, {"STEP"=0, "time[ms]"=250.0, "time tolerance[us]"=0.01, "CH0"=TRUE, "rel. amplitude CH0"=1.0, "phase [°] CH0"=0.0, "f0 [Hz] CH0"=81809301.07020178, "f1 [Hz] CH0"=81848283.63995752, "CH1"=FALSE, "rel. amplitude CH1"=1.0, "phase [°] CH1"=0.0, "f0 [Hz] CH1"=80000000.0, "f1 [Hz] CH1"=80000000.0}, {"STEP"=0, "time[ms]"=250.0, "time tolerance[us]"=0.01, "CH0"=TRUE, "rel. amplitude CH0"=1.0, "phase [°] CH0"=0.0, "f0 [Hz] CH0"=81848283.63995752, "f1 [Hz] CH0"=81879826.69965199, "CH1"=FALSE, "rel. amplitude CH1"=1.0, "phase [°] CH1"=0.0, "f0 [Hz] CH1"=80000000.0, "f1 [Hz] CH1"=80000000.0}, {"STEP"=0, "time[ms]"=250.0, "time tolerance[us]"=0.01, "CH0"=TRUE, "rel. amplitude CH0"=1.0, "phase [°] CH0"=0.0, "f0 [Hz] CH0"=81879826.69965199, "f1 [Hz] CH0"=81905148.25364487, "CH1"=FALSE, "rel. amplitude CH1"=1.0, "phase [°] CH1"=0.0, "f0 [Hz] CH1"=80000000.0, "f1 [Hz] CH1"=80000000.0}, {"STEP"=0, "time[ms]"=250.0, "time tolerance[us]"=0.01, "CH0"=TRUE, "rel. amplitude CH0"=1.0, "phase [°] CH0"=0.0, "f0 [Hz] CH0"=81905148.25364487, "f1 [Hz] CH0"=81925346.22531174, "CH1"=FALSE, "rel. amplitude CH1"=1.0, "phase [°] CH1"=0.0, "f0 [Hz] CH1"=80000000.0, "f1 [Hz] CH1"=80000000.0}, {"STEP"=0, "time[ms]"=250.0, "time tolerance[us]"=0.01, "CH0"=TRUE, "rel. amplitude CH0"=1.0, "phase [°] CH0"=0.0, "f0 [Hz] CH0"=81925346.22531174, "f1 [Hz] CH0"=81941375.53849728, "CH1"=FALSE, "rel. amplitude CH1"=1.0, "phase [°] CH1"=0.0, "f0 [Hz] CH1"=80000000.0, "f1 [Hz] CH1"=80000000.0}, {"STEP"=0, "time[ms]"=250.0, "time tolerance[us]"=0.01, "CH0"=TRUE, "rel. amplitude CH0"=1.0, "phase [°] CH0"=0.0, "f0 [Hz] CH0"=81941375.53849728, "f1 [Hz] CH0"=81954045.26017995, "CH1"=FALSE, "rel. amplitude CH1"=1.0, "phase [°] CH1"=0.0, "f0 [Hz] CH1"=80000000.0, "f1 [Hz] CH1"=80000000.0}, {"STEP"=0, "time[ms]"=250.0, "time tolerance[us]"=0.01, "CH0"=TRUE, "rel. amplitude CH0"=1.0, "phase [°] CH0"=0.0, "f0 [Hz] CH0"=81954045.26017995, "f1 [Hz] CH0"=81964027.58007582, "CH1"=FALSE, "rel. amplitude CH1"=1.0, "phase [°] CH1"=0.0, "f0 [Hz] CH1"=80000000.0, "f1 [Hz] CH1"=80000000.0}, {"STEP"=0, "time[ms]"=250.0, "time tolerance[us]"=0.01, "CH0"=TRUE, "rel. amplitude CH0"=1.0, "phase [°] CH0"=0.0, "f0 [Hz] CH0"=81964027.58007582, "f1 [Hz] CH0"=81971872.7459135, "CH1"=FALSE, "rel. amplitude CH1"=1.0, "phase [°] CH1"=0.0, "f0 [Hz] CH1"=80000000.0, "f1 [Hz] CH1"=80000000.0}, {"STEP"=0, "time[ms]"=250.0, "time tolerance[us]"=0.01, "CH0"=TRUE, "rel. amplitude CH0"=1.0, "phase [°] CH0"=0.0, "f0 [Hz] CH0"=81971872.7459135, "f1 [Hz] CH0"=81978026.1147388, "CH1"=FALSE, "rel. amplitude CH1"=1.0, "phase [°] CH1"=0.0, "f0 [Hz] CH1"=80000000.0, "f1 [Hz] CH1"=80000000.0}, {"STEP"=0, "time[ms]"=250.0, "time tolerance[us]"=0.01, "CH0"=TRUE, "rel. amplitude CH0"=1.0, "phase [°] CH0"=0.0, "f0 [Hz] CH0"=81978026.1147388, "f1 [Hz] CH0"=81982845.02917257, "CH1"=FALSE, "rel. amplitude CH1"=1.0, "phase [°] CH1"=0.0, "f0 [Hz] CH1"=80000000.0, "f1 [Hz] CH1"=80000000.0}, {"STEP"=0, "time[ms]"=250.0, "time tolerance[us]"=0.01, "CH0"=TRUE, "rel. amplitude CH0"=1.0, "phase [°] CH0"=0.0, "f0 [Hz] CH0"=81982845.02917257, "f1 [Hz] CH0"=81986614.29815143, "CH1"=FALSE, "rel. amplitude CH1"=1.0, "phase [°] CH1"=0.0, "f0 [Hz] CH1"=80000000.0, "f1 [Hz] CH1"=80000000.0}, {"STEP"=0, "time[ms]"=250.0, "time tolerance[us]"=0.01, "CH0"=TRUE, "rel. amplitude CH0"=1.0, "phase [°] CH0"=0.0, "f0 [Hz] CH0"=81986614.29815143, "f1 [Hz] CH0"=81989559.74861288, "CH1"=FALSE, "rel. amplitude CH1"=1.0, "phase [°] CH1"=0.0, "f0 [Hz] CH1"=80000000.0, "f1 [Hz] CH1"=80000000.0}]
  out "error out":errorcluster={"status"=TRUE, "code"=-1073807339, "source"="VISA Read in FlexDDS-NG_USB_Example.vi"}
  out "read buffer":string
  in  "FlexDDS-NG USB VISA resource name (COM)":refnum<visa-resource-name>="COM5"
  # "STEP"
  # "time [ms]"
  # "time tolerance [us]"
  # "CH0 [false=wait, keep phase&amplitude]"
  # "rel. amplitude CH0"
  # "phase [°] CH0"
  # "f0 [Hz] CH0"
  # "f1 [Hz] CH0"
  # "CH1 [false=wait, keep phase&amplitude]"
  # "rel. amplitude CH1"
  # "phase [°] CH1"
  # "f0 [Hz] CH1"
  # "f1 [Hz] CH1"
  # "f(t) = f0 + (f1-f0)/(1+exp(-k/Dt * (t-Dt/2)))"
  # "f(t) = f1 - (f1-f0)*exp(-K*t/Dt)"
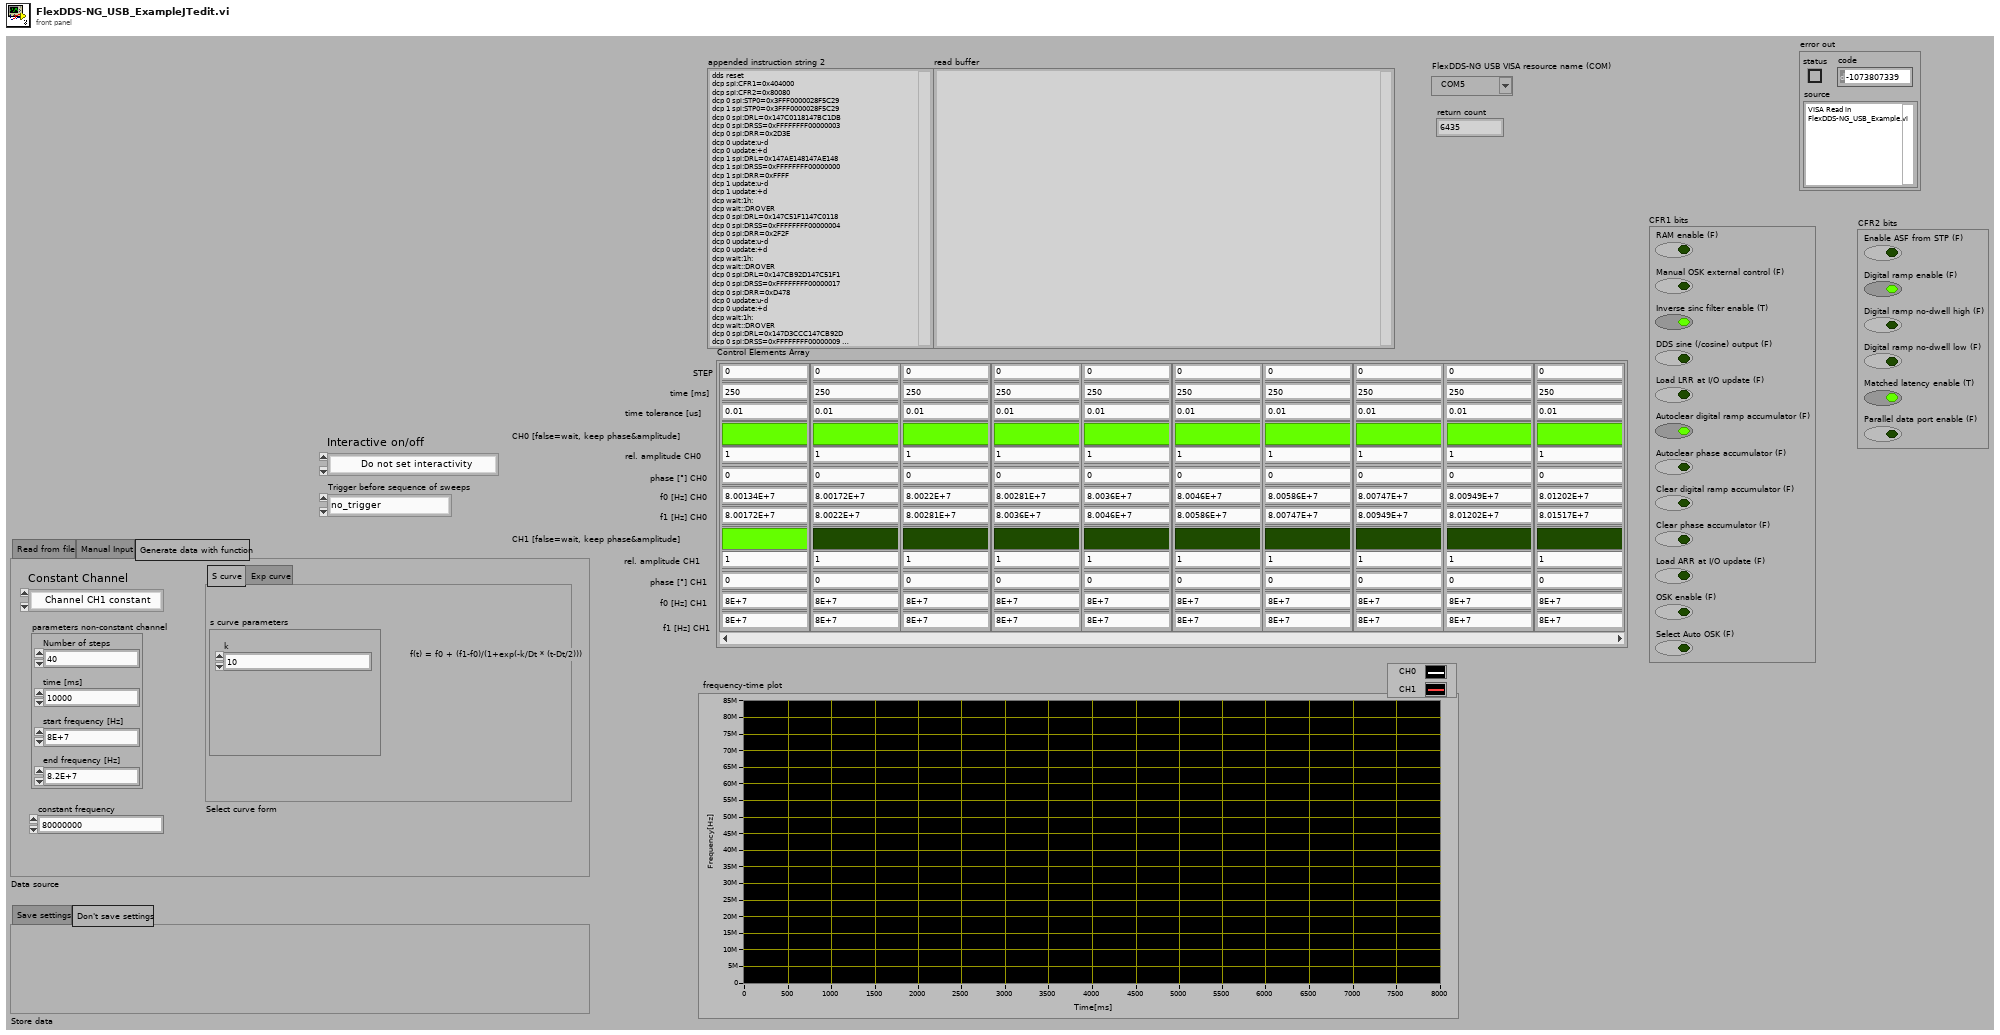
[diagram p1: front panel]
types:
  T1 = enum16{"Do not set interactivity", "Interactive off", "Interactive on"}
  T2 = enum32{"Read from file", "Manual Input", "Generate data with function"}
  T3 = cluster{"Number of steps":i32, "time [ms]":dbl, "start frequency [Hz]":dbl, "end frequency [Hz]":dbl}
  T4 = enum16{"Channel CH1 constant", "Channel CH0 constant"}
  T5 = cluster{"Enable ASF from STP (F)":bool, "Digital ramp enable (F)":bool, "Digital ramp no-dwell high (F)":bool, "Digital ramp no-dwell low (F)":bool, "Matched latency enable (T)":bool, "Parallel data port enable (F)":bool}
  T6 = cluster{"RAM enable (F)":bool, "Manual OSK external control (F)":bool, "Inverse sinc filter enable (T)":bool, "DDS sine (/cosine) output (F)":bool, "Load LRR at I/O update (F)":bool, "Autoclear digital ramp accumulator (F)":bool, "Autoclear phase accumulator (F)":bool, "Clear digital ramp accumulator (F)":bool, "Clear phase accumulator (F)":bool, "Load ARR at I/O update (F)":bool, "OSK enable (F)":bool, "Select Auto OSK (F)":bool}
  T7 = enum16{"no_trigger", "BNC_IN_A_RISING", "BNC_IN_A_FALLING", "BNC_IN_B_RISING", "BNC_IN_B_FALLING", "BNC_IN_C_RISING", "BNC_IN_C_FALLING"}
  T8 = cluster{cluster{"total time[ms]":dbl, "f1 [Hz] CH0":dbl}[]}[]
  T9 = cluster{"STEP":i32, "time[ms]":dbl, "time tolerance[us]":dbl, "CH0":bool, "rel. amplitude CH0":dbl, "phase [°] CH0":dbl, "f0 [Hz] CH0":dbl, "f1 [Hz] CH0":dbl, "CH1":bool, "rel. amplitude CH1":dbl, "phase [°] CH1":dbl, "f0 [Hz] CH1":dbl, "f1 [Hz] CH1":dbl}[]
  T10 = cluster{i32, dbl, "time tolerance":dbl, bool, dbl, dbl, "constant frequency":dbl, "constant frequency":dbl, bool, dbl, dbl, "constant frequency":dbl, "constant frequency":dbl}[]
  T11 = cluster{i32, dbl, "time tolerance":dbl, bool, dbl, dbl, "constant frequency":dbl, "constant frequency":dbl, bool, dbl, dbl, "constant frequency":dbl, "constant frequency":dbl}
  T12 = cluster{"total time[ms]":dbl, "f1 [Hz] CH1":dbl}[]
  T13 = cluster{"total time[ms]":dbl, "f1 [Hz] CH0":dbl}[]
  T14 = cluster{"STEP":i32, "time[ms]":dbl, "time tolerance[us]":dbl, "CH0":bool, "rel. amplitude CH0":dbl, "phase [°] CH0":dbl, "f0 [Hz] CH0":dbl, "f1 [Hz] CH0":dbl, "CH1":bool, "rel. amplitude CH1":dbl, "phase [°] CH1":dbl, "f0 [Hz] CH1":dbl, "f1 [Hz] CH1":dbl}
  T15 = cluster{"Array":cluster{"total time[ms]":dbl, "f1 [Hz] CH0":dbl}[]}
  T16 = cluster{"Array":cluster{"total time[ms]":dbl, "f1 [Hz] CH1":dbl}[]}
  T17 = cluster{"Array":cluster{"total time[ms]":dbl, "f1 [Hz] CH1":dbl}[]}[]
  T18 = enum32{"Channel 0", "Channel 1", "Both channels"}
  T19 = enum32{"O_RAMP_SWP_OVR", "RAM_SWP_OVR", "O_DROVER", "DROVER", "O_SPI_FIFO_EV1", "SPI_FIFO_EV1", "O_SPI_FIFO_EV0", "SPI_FIFO_EV0", "O_SPI_FIFO_FLUSHED", "SPI_FIFO_FLUSHED", "BNC_IN_B_LEVEL", "BNC_IN_B_FALLING", "BNC_IN_B_RISING", "BNC_IN_A_LEVEL", "BNC_IN_A_FALLING", "BNC_IN_A_RISING", "ALL_SPI_FIFOS_FLUSHED", "NONE"}
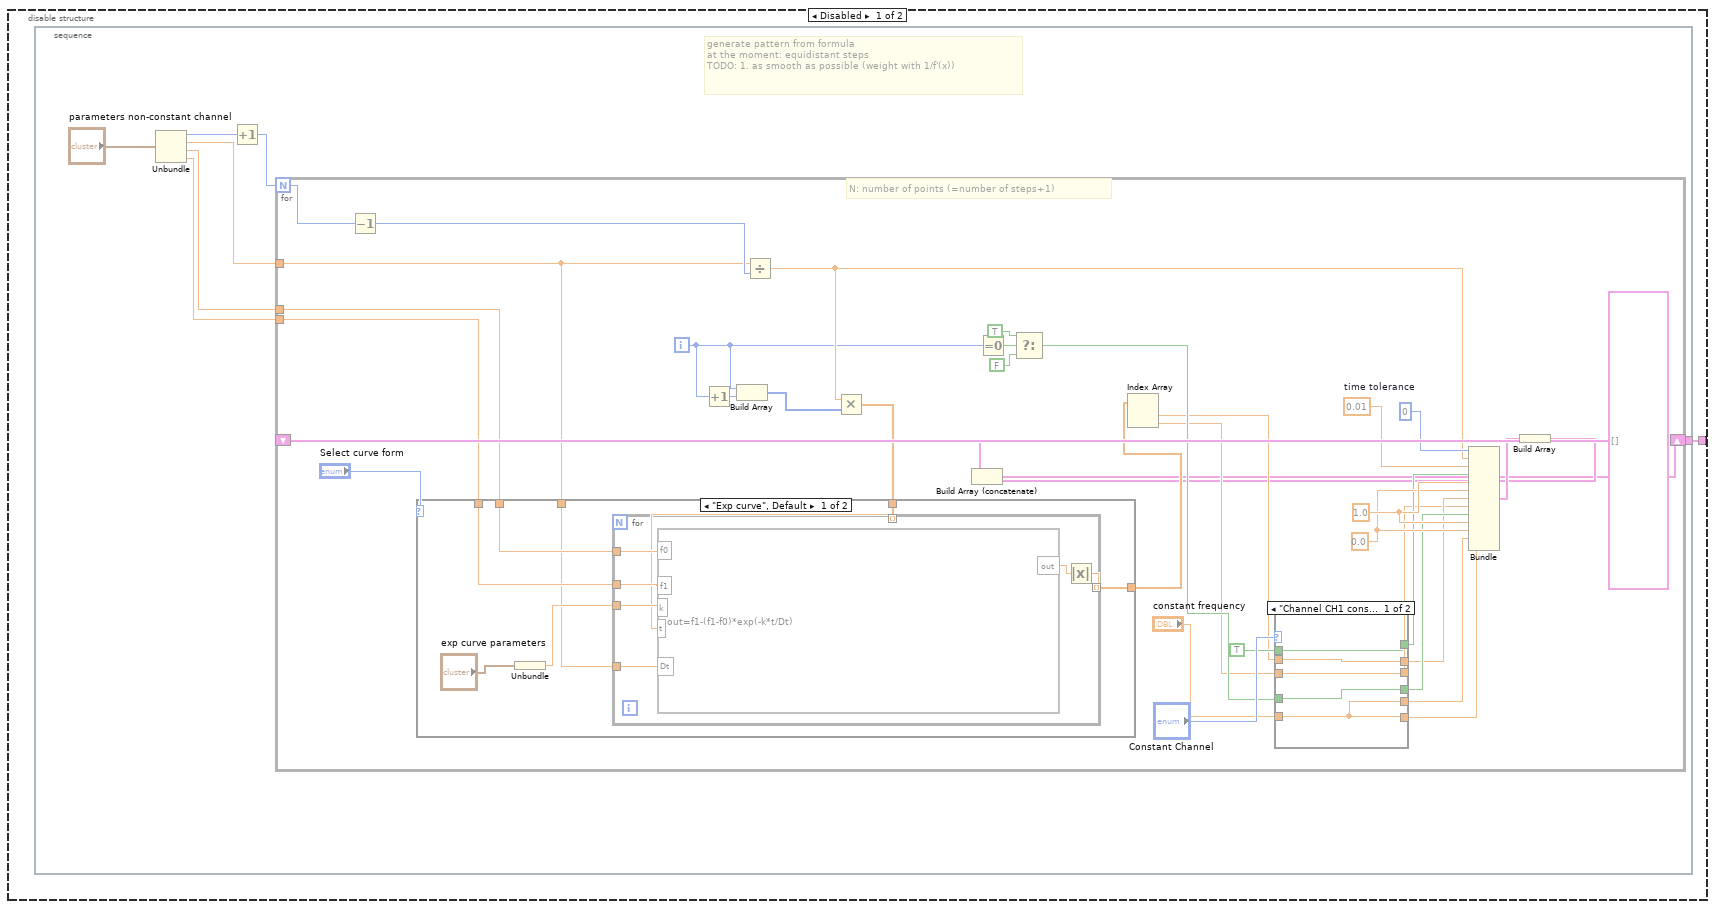
[diagram p2: hidden frame]
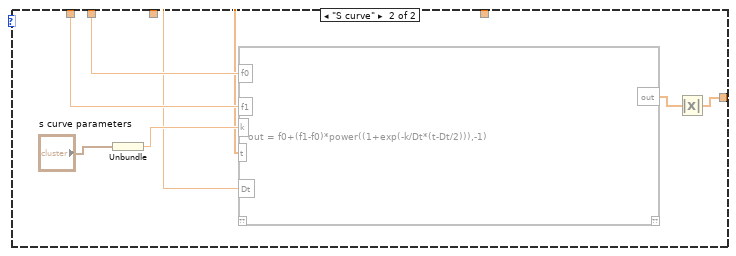
[diagram p4: hidden frame]
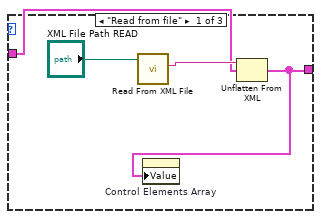
[diagram p5: hidden frame]
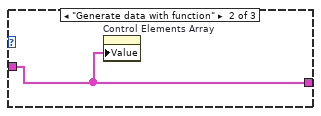
[diagram p6: hidden frame]
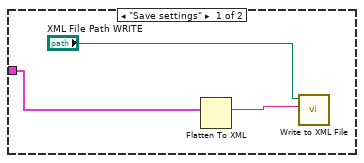
[diagram p7: hidden frame]
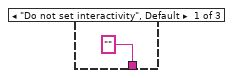
[diagram p10: hidden frame]
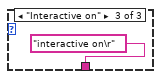
[diagram p11: hidden frame]
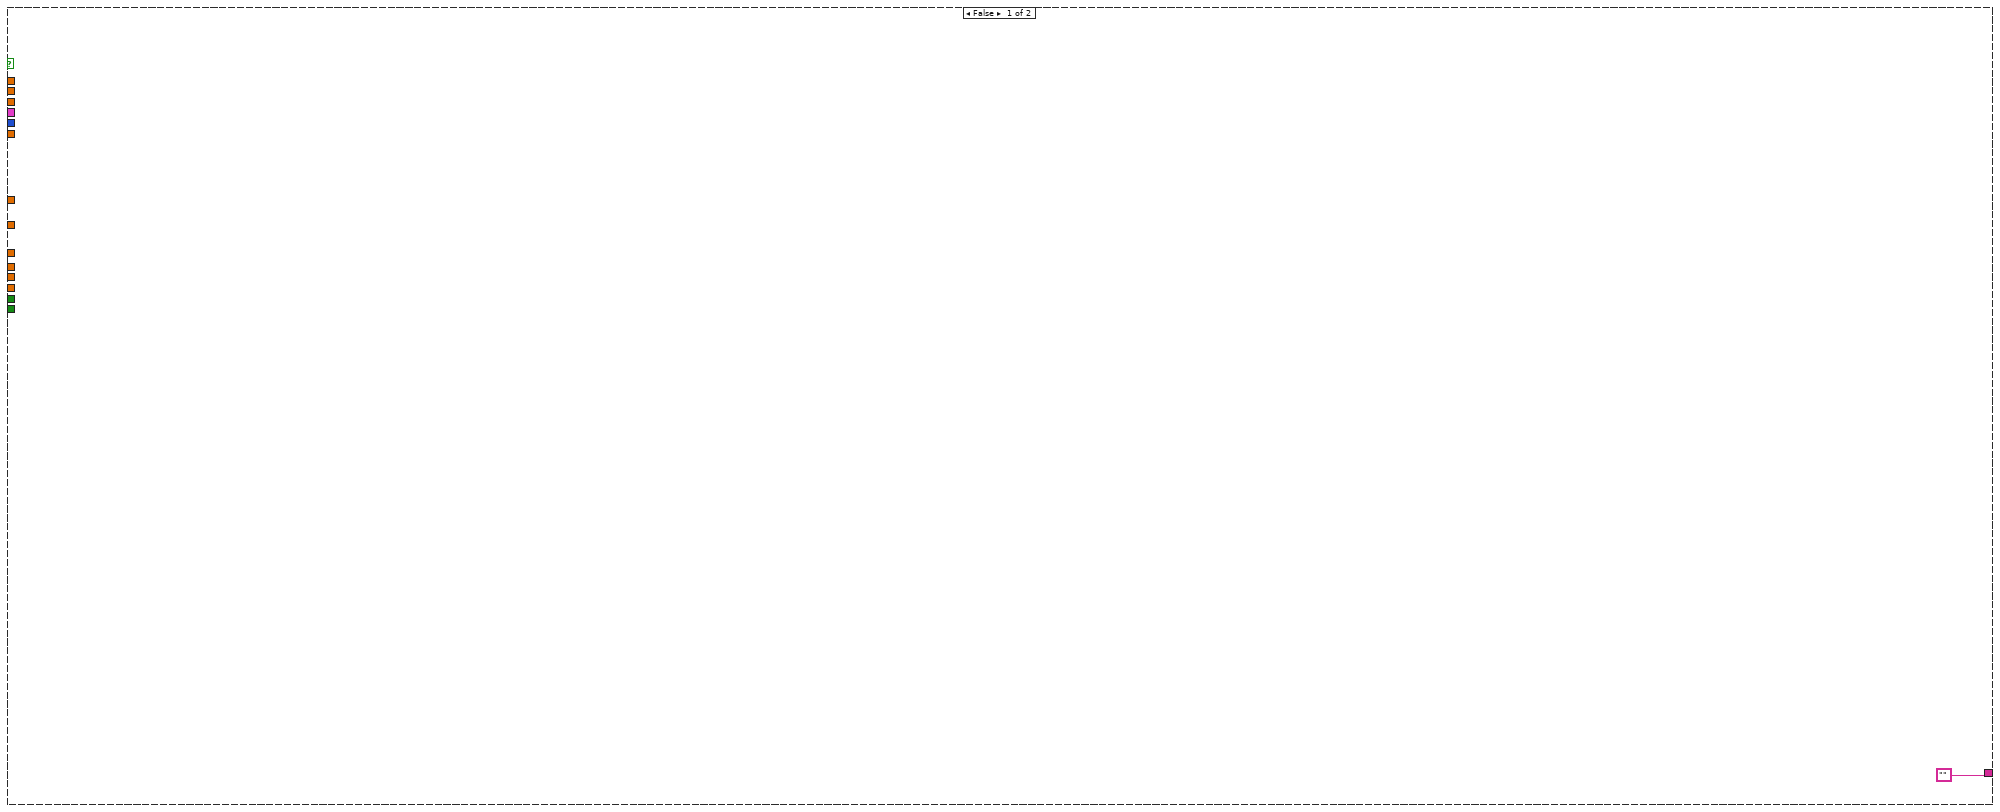
[diagram p12: hidden frame]
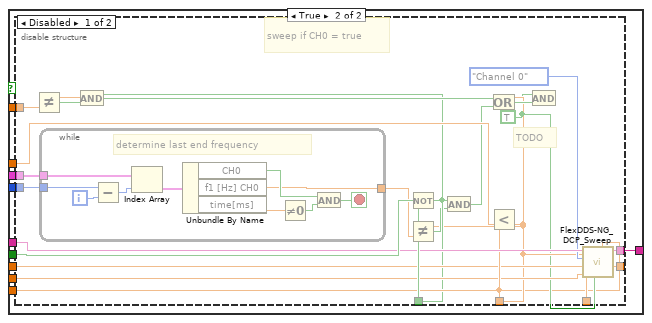
[diagram p15: hidden frame]
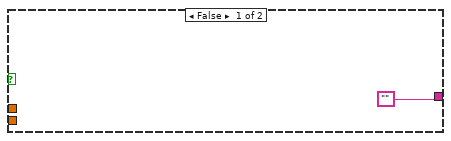
[diagram p18: hidden frame]
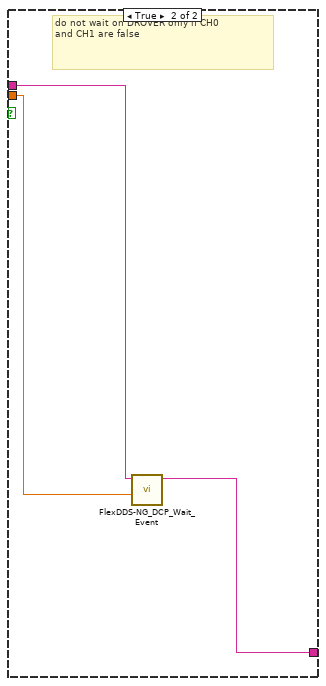
[diagram p19: hidden frame]
diagram:
  # "Relevant subvis for 'high level use':\nDCP Reset\nDCP Write STP\nDCP Write CFR1\nDCP Write CFR2\nDCP Write DRL\nDCP Write DRR\nDCP CMD (Bool)\nDCP Wait BNC\nDCP Wait Event\nDCP Start Stop\nTime To M/P\nDCP Sweep"
  n1 = disable-structure shown="Enabled" {
    disable-tunnel: [w23 _] -> w14
    frame Disabled {
      n2 = stacked-sequence {
        tunnel: [w30] -> w23
        frame #0 {
          # "generate pattern from formula\nat the moment: equidistant steps\nTODO: 1. as smooth as possible (weight with 1/f'(x))"
          n3 = Unbundle("parameters non-constant channel") -> ("Number of steps"=w29:i32, "time [ms]"=w27:dbl, "start frequency [Hz]"=w26:dbl, "end frequency [Hz]"=w25:dbl)
          n4 = Increment(x=w29) -> (x+1=w31:i32)
          n5 = for {
            N: w31 -> [w60]
            tunnel: w27 -> [w48]
            tunnel: w26 -> [w57]
            tunnel: w25 -> [w58]
            shift-right: [w32] -> w30
            shift-left: T10 [] -> [w33]
            i -> [w51]
            w63 = 1.0
            w62 = 0.0
            w64 = 0.01  # time tolerance
            # "N: number of points (=number of steps+1)"
            n6 = Decrement(x=w60) -> (x-1=w59:i32)
            n7 = Increment(x=w51) -> (x+1=w50:i32)
            n8 = Build Array(w51, w50) -> (w49:i32[])
            n9 = Divide(x=w48, y=w59) -> (x/y=w55:dbl)
            n10 = Multiply(x=w55, y=w49) -> (x*y=w56:dbl[])
            n11 = case shown="\"Exp curve\", Default" "Select curve form" {
              tunnel: w58 -> [w81 w96]
              tunnel: w57 -> [w82 w97]
              tunnel: w56 -> [w79 w94]
              tunnel: w48 -> [w78 w93]
              tunnel: [w77 w91] -> w47
              frame "Exp curve", Default {
                n12 = Unbundle("exp curve parameters") -> ("k"=w80:dbl)
                n13 = for {
                  tunnel: w82 -> [w90]
                  tunnel: w81 -> [w89]
                  tunnel: w80 -> [w88]
                  tunnel: w79 -> [w87] mode=indexing
                  tunnel: w78 -> [w86]
                  tunnel: [w84] -> w77 mode=indexing
                  n14 = formula code="out=f1-(f1-f0)*exp(-k*t/Dt)"("f0"=w90, "f1"=w89, "k"=w88, "t"=w87, "Dt"=w86) -> ("out"=w85:dbl)
                  n15 = Absolute Value(x=w85) -> (abs(x)=w84:dbl)
                }
              }
              frame "S curve" {
                n16 = Unbundle("s curve parameters") -> ("k"=w95:dbl)
                n17 = mathscript code="out = f0+(f1-f0)*power((1+exp(-k/Dt*(t-Dt/2))),-1)"("f0"=w97, "f1"=w96, "k"=w95, "t"=w94, "Dt"=w93) -> ("out"=w92:cdb[])  [unwired: 1 in, 1 out]
                n18 = Absolute Value(x=w92) -> (abs(x)=w91:dbl[])
              }
            }
            n19 = Equal To 0?(x=w51) -> (x = 0?=w54:bool)
            n20 = Select(t=TRUE, s=w54, f=FALSE) -> (s? t:f=w42:bool)
            n21 = Index Array(array=w47) -> (element #1=w38:dbl, element #2=w37:dbl)  [unwired: 2 in]
            n22 = case shown="\"Channel CH1 constant\", Default" "Constant Channel" {
              tunnel: "constant frequency" -> [w71 w72]
              tunnel: [w71 w74] -> w44
              tunnel: [w71 w75] -> w43
              tunnel: w42 -> [w70 w73]
              tunnel: [w70 w76] -> w41
              tunnel: TRUE -> [w69 w76]
              tunnel: [w69 w73] -> w39
              tunnel: w38 -> [w68 w75]
              tunnel: w37 -> [w67 w74]
              tunnel: [w68 w72] -> w36
              tunnel: [w67 w72] -> w35
              frame "Channel CH1 constant", Default {
              }
              frame "Channel CH0 constant" {
              }
            }
            n23 = Bundle(0, w55, "time tolerance"=w64, w39, w63, w62, "constant frequency"=w36, "constant frequency"=w35, w41, w63, w62, "constant frequency"=w43, "constant frequency"=w44) -> (w66:T11)  [unwired: 1 in]
            n24 = Build Array(w66) -> (w34:T10)
            n25 = Build Array (concatenate)(w33, w34) -> (w32:T10)
          }
        }
      }
    }
    frame Enabled {
    }
  }
  n26 = flat-sequence {
    tunnel: w14 -> [w99]
    tunnel: [w100] -> w13
    tunnel: w13 -> [w109]
    tunnel: [w109] -> w12
    tunnel: w12 -> [w116]
    tunnel: [w116] -> w11
    frame #0 {
      # "Input: read settings from xml file\nor generate data with function\nor use manual input from array"
      n27 = case shown="\"Manual Input\"" "Data source" {
        tunnel: w99 -> [w103 w106 _]
        tunnel: [w102 w106 w107] -> w100
        frame "Read from file" {
          n28 = call-poly <vilib>:"Read From XML File.vi"("XML File Path"="XML File Path READ") -> ("XML Elements"=w104:string)  [unwired: 8 in, 2 out]
          n29 = Unflatten From XML(xml string=w104, type=w103) -> (value=w102:T10)  [unwired: 1 in, 1 out]
          n30 = property on="Control Elements Array" class="Arr (strict)"("Value"=w102) -> ()  [unwired: 2 in, 2 out]
        }
        frame "Generate data with function" {
          n31 = property on="Control Elements Array" class="Arr (strict)"("Value"=w106) -> ()  [unwired: 2 in, 2 out]
        }
        frame "Manual Input" {
          n32 = property on="Control Elements Array" class="Arr (strict)"() -> ("Value"=w107:T9)  [unwired: 2 in, 2 out]
        }
      }
    }
    frame #1 {
      # "save array/settings or don't save anything"
      n33 = case shown="\"Don't save settings\", Default" "Store data" {
        tunnel: w109 -> [w110 _]
        frame "Save settings" {
          n34 = Flatten To XML(anything=w110) -> (xml string=w112:string)
          n35 = call-poly <vilib>:"Write to XML File.vi"("XML Input"=w112, "XML File Path"="XML File Path WRITE") -> ()  [unwired: 7 in, 3 out]
        }
        frame "Don't save settings", Default {
        }
      }
    }
    frame #2 {
      w117 = 0.0  # total time[ms]
      # "plot frequency time plot AFTER reading"
      n36 = for {
        N: 5 -> [_]
        tunnel: w116 -> [w151] mode=indexing
        shift-right: [w150] -> _
        shift-left: w117 -> [w146]
        tunnel: w116 -> [w147]
        shift-right: [w125] -> w121
        shift-left: T13 [] ("Array") -> [w126]
        shift-right: [w123] -> w122
        shift-left: T12 [] ("Array") -> [w124]
        i -> [w148]
        # "iterate through linear ramps;\nif time==0: skip;\nif CHx==false: keep frequency;"
        n37 = flat-sequence {
          tunnel: w148 -> [w161]
          tunnel: w147 -> [w162]
          tunnel: [w163] -> w135
          tunnel: [w160] -> w134
          frame #0 {
            # "i: current index\nif CHx == false, look for largest index j<i with CHx=true (to determine which frequency to plot)"
            n38 = while {
              tunnel: w161 -> [w183]
              tunnel: w162 -> [w180]
              tunnel: [w178] -> w163
              i -> [w182]
              stop <- w176 stop-if-true
              n39 = Subtract(x=w183, y=w182) -> (x-y=w181:i32)
              n40 = Index Array(array=w180, index=w181) -> (element=w179:T14)
              n41 = Unbundle By Name(w179) -> ("f1 [Hz] CH0"=w178:dbl, "CH0"=w175:bool, "time[ms]"=w177:dbl)
              n42 = Not Equal To 0?(x=w177) -> (x != 0?=w174:bool)
              n43 = And(x=w175, y=w174) -> (x .and. y?=w176:bool)
            }
            n44 = while {
              tunnel: w161 -> [w173]
              tunnel: w162 -> [w170]
              tunnel: [w168] -> w160
              i -> [w172]
              stop <- w166 stop-if-true
              n45 = Subtract(x=w173, y=w172) -> (x-y=w171:i32)
              n46 = Index Array(array=w170, index=w171) -> (element=w169:T14)
              n47 = Unbundle By Name(w169) -> ("f1 [Hz] CH1"=w168:dbl, "CH1"=w165:bool, "time[ms]"=w167:dbl)
              n48 = Not Equal To 0?(x=w167) -> (x != 0?=w164:bool)
              n49 = And(x=w165, y=w164) -> (x .and. y?=w166:bool)
            }
          }
        }
        n50 = Unbundle By Name(w151) -> ("time[ms]"=w149:dbl, "f0 [Hz] CH0"=w139:dbl, "f1 [Hz] CH0"=w138:dbl, "f0 [Hz] CH1"=w137:dbl, "f1 [Hz] CH1"=w136:dbl, "CH0"=w141:bool, "CH1"=w140:bool)
        n51 = Add(x=w146, y=w149) -> (x+y=w150:dbl)
        n52 = Not Equal To 0?(x=w149) -> (x != 0?=w127:bool)
        n53 = Select(t=w139, s=w141, f=w135) -> (s? t:f=w143:dbl)
        n54 = Select(t=w138, s=w141, f=w135) -> (s? t:f=w142:dbl)
        n55 = Select(t=w137, s=w140, f=w134) -> (s? t:f=w145:dbl)
        n56 = Select(t=w136, s=w140, f=w134) -> (s? t:f=w144:dbl)
        n57 = Bundle("total time[ms]"=w146, "f1 [Hz] CH0"=w143) -> (w133:cluster{"total time[ms]":dbl, "f1 [Hz] CH0":dbl})  [unwired: 1 in]
        n58 = Bundle(w150, "f1 [Hz] CH0"=w142) -> (w132:cluster{dbl, "f1 [Hz] CH0":dbl})  [unwired: 1 in]
        n59 = Bundle("total time[ms]"=w146, "f1 [Hz] CH1"=w145) -> (w131:cluster{"total time[ms]":dbl, "f1 [Hz] CH1":dbl})  [unwired: 1 in]
        n60 = Bundle(w150, "f1 [Hz] CH1"=w144) -> (w130:cluster{dbl, "f1 [Hz] CH1":dbl})  [unwired: 1 in]
        n61 = Build Array(w133, w132) -> (w129:T13)
        n62 = case shown="True" w127 {
          tunnel: w126 -> [w156 w158]
          tunnel: w129 -> [_ w157]
          tunnel: [w156 w159] -> w125
          frame False {
          }
          frame True {
            n63 = Build Array (concatenate)(w158, w157) -> (w159:T13)
          }
        }
        n64 = Build Array(w131, w130) -> (w128:T12)
        n65 = case shown="True" w127 {
          tunnel: w124 -> [w152 w154]
          tunnel: w128 -> [_ w153]
          tunnel: [w152 w155] -> w123
          frame False {
          }
          frame True {
            n66 = Build Array (concatenate)(w154, w153) -> (w155:T12)
          }
        }
      }
      n67 = Bundle("Array"=w121) -> (w118:T15)  [unwired: 1 in]
      n68 = Bundle("Array"=w122) -> (w119:T16)  [unwired: 1 in]
      n69 = Build Array(w118, w119) -> (→"frequency-time plot":T17)
    }
  }
  n70 = flat-sequence {
    frame #0 {
      # "This is the central data structure, work with property nodes to simplify reading and writing settings"
    }
  }
  n71 = flat-sequence {
    tunnel: [w189] -> w21
    tunnel: [w187] -> w20
    tunnel: w11 -> [w187]
    tunnel: w21 -> [w198]
    tunnel: w20 -> [w193]
    tunnel: [w196] -> w18
    tunnel: [w193] -> w16
    tunnel: w18 -> [w201]
    tunnel: [w200] -> w17
    tunnel: w16 -> [w204]
    tunnel: [w204] -> w15
    tunnel: w17 -> [w205]
    tunnel: w15 -> [w209]
    tunnel: [w207] -> w19
    tunnel: [w456] -> w22
    tunnel: w19 -> [w455]
    frame #0 {
      # "Interactive off + Full Reset"
      n72 = case shown="\"Interactive off\"" "Interactive on/off" {
        tunnel: ["" ("input 1") "interactive off\r" ("input 1") "interactive on\r" ("input 1")] -> w184
        frame "Do not set interactivity", Default {
        }
        frame "Interactive off" {
        }
        frame "Interactive on" {
        }
      }
      n73 = Format Into String(w184) -> (resulting string=w186:string)  [unwired: 3 in, 1 out]
      n74 = call "FlexDDS-NG_DCP_Reset.vi"("full reset (yes)"=TRUE, "initial instruction string"=w186) -> ("appended instruction string"=w189:string)  [unwired: 9 in]
    }
    frame #1 {
      w197 = T18."Both channels" ("Channels")
      # "* inverse sinc filter\n* digital ramp enable\n* matched latency enable"
      # "Write CFR1 and CFR2"
      n75 = call "FlexDDS-NG_DCP_WriteCFR1_C.vi"("CFR1 bits"="CFR1 bits", "Channels"=w197, "initial instruction string"=w198) -> ("appended instruction string"=w199:string)  [unwired: 8 in]
      n76 = call "FlexDDS-NG_DCP_WriteCFR2_C.vi"("CFR2 bits"="CFR2 bits", "Channels"=w197, "initial instruction string"=w199) -> ("appended instruction string"=w196:string)  [unwired: 8 in]
    }
    frame #2 {
      # "add trigger"
      n77 = call "FlexDDS-NG_DCP_Wait_BNC.vi"("Trigger"="Trigger before sequence of sweeps", "Channels"=T18."Both channels" ("Channels 2"), "appended instruction string in"=w201) -> ("appended instruction string"=w200:string)  [unwired: 8 in]
    }
    frame #3 {
      # "iterate through array of clusters and create command string\nif 1st command is decreasing ramp add very short increasing ramp before\nignore all columns with time=0ms\nTODO: write some detailed documentation what is going on below"
      n78 = Array Size(array=w209) -> (size(s)=w210:i32)
      n79 = for {
        N: w210 -> [_]
        tunnel: w209 -> [w240] mode=indexing
        tunnel: w209 -> [w226]
        tunnel: [w239] -> w208 mode=indexing
        i -> [w238]
        # "iterate through array of time steps"
        n80 = Unbundle(w240) -> ("time[ms]"=w232:dbl, "time tolerance[us]"=w231:dbl, "CH0"=w237:bool, "rel. amplitude CH0"=w230:dbl, "phase [°] CH0"=w229:dbl, "f0 [Hz] CH0"=w236:dbl, "f1 [Hz] CH0"=w235:dbl, "CH1"=w211:bool, "rel. amplitude CH1"=w228:dbl, "phase [°] CH1"=w227:dbl, "f0 [Hz] CH1"=w234:dbl, "f1 [Hz] CH1"=w233:dbl)  [unwired: 1 out]
        n81 = flat-sequence {
          tunnel: w226 -> [w288]
          tunnel: w227 -> [w252]
          tunnel: w228 -> [w253]
          tunnel: w229 -> [w256]
          tunnel: w230 -> [w257]
          tunnel: w231 -> [w289]
          tunnel: w232 -> [w243]
          tunnel: w233 -> [w250]
          tunnel: w234 -> [w251]
          tunnel: w235 -> [w254]
          tunnel: w236 -> [w255]
          tunnel: w237 -> [w261]
          tunnel: w238 -> [w248]
          tunnel: [w248] -> w225
          tunnel: [w261] -> w224
          tunnel: [w258] -> w223
          tunnel: [w255] -> w222
          tunnel: [w254] -> w221
          tunnel: [w251] -> w220
          tunnel: [w250] -> w219
          tunnel: [w243] -> w218
          tunnel: [w289] -> w217
          tunnel: [w257] -> w216
          tunnel: [w256] -> w215
          tunnel: [w253] -> w214
          tunnel: [w252] -> w213
          tunnel: [w288] -> w212
          tunnel: w211 -> [w258]
          tunnel: [w304] -> w239
          tunnel: w225 -> [w303]
          tunnel: w224 -> [w302]
          tunnel: w223 -> [w301]
          tunnel: w222 -> [w291]
          tunnel: w221 -> [w290]
          tunnel: w220 -> [w300]
          tunnel: w219 -> [w299]
          tunnel: w218 -> [w298]
          tunnel: w217 -> [w292]
          tunnel: w216 -> [w297]
          tunnel: w215 -> [w296]
          tunnel: w214 -> [w295]
          tunnel: w213 -> [w294]
          tunnel: w212 -> [w293]
          frame #0 {
            # "0<=ampl<=1\n0<=freq<=400MHz\n0<=phase=360\nChx[0] not FALSE\ntime[0] not 0"
            # "check if input is valid\nabort otherwise"
            n82 = Equal To 0?(x=w248) -> (x = 0?=w245:bool)
            n83 = Equal To 0?(x=w243) -> (x = 0?=w244:bool)
            n84 = In Range and Coerce(upper limit=360.0, x=w256, lower limit=0.0) -> (In Range?=w268:bool)  [unwired: 1 out]
            n85 = In Range and Coerce(upper limit=360.0, x=w252, lower limit=0.0) -> (In Range?=w267:bool)  [unwired: 1 out]
            n86 = And(x=w245, y=w244) -> (x .and. y?=w242:bool)
            n87 = Not(x=w242) -> (.not. x?=w241:bool)
            n88 = Select(t=w261, s=w245, f=TRUE) -> (s? t:f=w263:bool)
            n89 = Select(t=w258, s=w245, f=TRUE) -> (s? t:f=w259:bool)
            n90 = In Range and Coerce(upper limit=400000000.0, x=w255, lower limit=0.0) -> (In Range?=w272:bool)  [unwired: 1 out]
            n91 = In Range and Coerce(upper limit=400000000.0, x=w254, lower limit=0.0) -> (In Range?=w271:bool)  [unwired: 1 out]
            n92 = In Range and Coerce(upper limit=400000000.0, x=w251, lower limit=0.0) -> (In Range?=w270:bool)  [unwired: 1 out]
            n93 = In Range and Coerce(upper limit=400000000.0, x=w250, lower limit=0.0) -> (In Range?=w269:bool)  [unwired: 1 out]
            n94 = In Range and Coerce(upper limit=1.0, x=w257, lower limit=0.0) -> (In Range?=w266:bool)  [unwired: 1 out]
            n95 = In Range and Coerce(upper limit=1.0, x=w253, lower limit=0.0) -> (In Range?=w265:bool)  [unwired: 1 out]
            n96 = Compound Arithmetic op=AND(w272, w271, w270, w269, w268, w267, w266, w265, w263, w259, w241) -> (w249:bool)
            n97 = Not(x=w249) -> (.not. x?=w247:bool)
            n98 = call "Display Message to User"("Enable"=w247) -> ("OK"=w246:bool)  [unwired: 9 in, 1 out]
            n99 = Stop(stop? (T)=w246) -> ()
          }
          frame #1 {
            n100 = Not Equal?(x=0.0, y=w298) -> (x != y?=w305:bool)
            n101 = case shown="True" w305 {
              tunnel: ["" w349] -> w304
              tunnel: w303 -> [_ w315]
              tunnel: w302 -> [_ w326]
              tunnel: w301 -> [_ w318]
              tunnel: w298 -> [_ w310]
              tunnel: w300 -> [_ w317]
              tunnel: w299 -> [_ w308]
              tunnel: w297 -> [_ w330]
              tunnel: w296 -> [_ w338]
              tunnel: w295 -> [_ w337]
              tunnel: w294 -> [_ w336]
              tunnel: w293 -> [_ w316]
              tunnel: w292 -> [_ w309]
              tunnel: w291 -> [_ w323]
              tunnel: w290 -> [_ w322]
              frame False {
              }
              frame True {
                # "1st iteration and amplitude or phase changed"
                # "skip if time is zero"
                n102 = Decrement(x=w315) -> (x-1=w348:i32)
                n103 = Not(x=w326) -> (.not. x?=w351:bool)
                n104 = Not(x=w318) -> (.not. x?=w350:bool)
                n105 = And(x=w351, y=w350) -> (x .and. y?=w352:bool)
                n106 = Index Array(array=w316, index=w348) -> (element=w321:T14)
                n107 = Unbundle By Name(w321) -> ("rel. amplitude CH0"=w344:dbl, "phase [°] CH0"=w343:dbl, "rel. amplitude CH1"=w340:dbl, "phase [°] CH1"=w339:dbl)
                n108 = Unbundle By Name(w321) -> ("CH0"=w319:bool, "CH1"=w312:bool, "f1 [Hz] CH0"=w320:dbl, "f1 [Hz] CH1"=w311:dbl)
                n109 = Equal?(x=w330, y=w344) -> (x = y?=w345:bool)
                n110 = Equal?(x=w338, y=w343) -> (x = y?=w346:bool)
                n111 = Equal?(x=w340, y=w337) -> (x = y?=w342:bool)
                n112 = And(x=w345, y=w346) -> (x .and. y?=w334:bool)
                n113 = Not(x=w334) -> (.not. x?=w333:bool)
                n114 = Equal To 0?(x=w315) -> (x = 0?=w347:bool)
                n115 = Or(x=w347, y=w333) -> (x .or. y?=w327:bool)
                n116 = And(x=w326, y=w327) -> (x .and. y?=w324:bool)
                n117 = case shown="True" w324 {
                  tunnel: w330 -> [_ w443]
                  tunnel: w338 -> [_ w442]
                  tunnel: ["" w441] -> w335
                  frame False {
                  }
                  frame True {
                    # "CH0: write stp if (i==0 or ampl/phase changed) and CH0 = true"
                    n118 = call "FlexDDS-NG_DCP_WriteSTP.vi"("phase degrees (0..360)"=w442, "amplitude (0..1)"=w443, "Channels"=T18."Channel 0", "initial instruction string"="") -> ("appended instruction string"=w441:string)  [unwired: 7 in]
                  }
                }
                n119 = Equal?(x=w339, y=w336) -> (x = y?=w341:bool)
                n120 = And(x=w342, y=w341) -> (x .and. y?=w332:bool)
                n121 = Not(x=w332) -> (.not. x?=w331:bool)
                n122 = Or(x=w347, y=w331) -> (x .or. y?=w328:bool)
                n123 = And(x=w318, y=w328) -> (x .and. y?=w325:bool)
                n124 = case shown="True" w325 {
                  tunnel: [w433 w438] -> w329
                  tunnel: w337 -> [_ w436]
                  tunnel: w336 -> [_ w435]
                  tunnel: w335 -> [w433 w434]
                  frame False {
                  }
                  frame True {
                    # "CH1: write stp if (i==0 or ampl/phase changed) and CH1 = true"
                    n125 = call "FlexDDS-NG_DCP_WriteSTP.vi"("phase degrees (0..360)"=w435, "amplitude (0..1)"=w436, "Channels"=T18."Channel 1", "initial instruction string"=w434) -> ("appended instruction string"=w438:string)  [unwired: 7 in]
                  }
                }
                n126 = case shown="False" w326 {
                  tunnel: w329 -> [w393 w399]
                  tunnel: [w393 w398] -> w314
                  tunnel: w310 -> [_ w396]
                  tunnel: w309 -> [_ w395]
                  tunnel: w323 -> [_ w397]
                  tunnel: w322 -> [_ w394]
                  tunnel: w320 -> [_ w403]
                  tunnel: w319 -> [_ w402]
                  tunnel: w316 -> [_ w401]
                  tunnel: w315 -> [_ w400]
                  frame False {
                  }
                  frame True {
                    n127 = disable-structure shown="Disabled" {
                      disable-tunnel: w403 -> [w421 _]
                      disable-tunnel: w402 -> [w416 _]
                      disable-tunnel: w401 -> [w414 _]
                      disable-tunnel: w400 -> [w413 _]
                      disable-tunnel: w399 -> [w410 _]
                      disable-tunnel: [w409 _] -> w398
                      disable-tunnel: w397 -> [w408 _]
                      disable-tunnel: w396 -> [w407 _]
                      disable-tunnel: w395 -> [w406 _]
                      disable-tunnel: w394 -> [w404 _]
                      frame Disabled {
                        w405 = TRUE ("x")
                        # "TODO"
                        # "sweep if CH0 = true"
                        n128 = Not Equal?(x=w408, y=w421) -> (x != y?=w419:bool)
                        n129 = while {
                          tunnel: w414 -> [w432]
                          tunnel: w413 -> [w430]
                          tunnel: [w423] -> w412
                          i -> [w431]
                          stop <- w424 stop-if-true
                          # "determine last end frequency"
                          n130 = Subtract(x=w430, y=w431) -> (x-y=w429:i32)
                          n131 = Index Array(array=w432, index=w429) -> (element=w428:T14)
                          n132 = Unbundle By Name(w428) -> ("CH0"=w425:bool, "f1 [Hz] CH0"=w423:dbl, "time[ms]"=w427:dbl)
                          n133 = Not Equal To 0?(x=w427) -> (x != 0?=w426:bool)
                          n134 = And(x=w425, y=w426) -> (x .and. y?=w424:bool)
                        }
                        n135 = And(x=w416, y=w419) -> (x .and. y?=w420:bool)
                        n136 = Not(x=w416) -> (.not. x?=w417:bool)
                        n137 = Not Equal?(x=w408, y=w412) -> (x != y?=w415:bool)
                        n138 = And(x=w417, y=w415) -> (x .and. y?=w418:bool)
                        n139 = Or(x=w420, y=w418) -> (x .or. y?=w422:bool)
                        n140 = Less?(x=w404, y=w408) -> ()  [unwired: 1 out]
                        n141 = And(x=w405, y=w422) -> ()  [unwired: 1 out]
                        n142 = call "FlexDDS-NG_DCP_Sweep.vi"("f1"=w404, "jump before ramp"=w405, "f0"=w408, "sweep time tolerance (us)"=w406, "sweep time (ms)"=w407, "Channels in"=T18."Channel 0", "initial instruction string"=w410) -> ("appended instruction string out"=w409:string)  [unwired: 4 in]
                      }
                      frame Enabled {
                      }
                    }
                  }
                }
                n143 = case shown="True" w318 {
                  tunnel: w314 -> [w353 w358]
                  tunnel: [w353 w357] -> w313
                  tunnel: w310 -> [_ w355]
                  tunnel: w309 -> [_ w354]
                  tunnel: w317 -> [_ w356]
                  tunnel: w308 -> [_ w359]
                  tunnel: w311 -> [_ w363]
                  tunnel: w312 -> [_ w362]
                  tunnel: w316 -> [_ w361]
                  tunnel: w315 -> [_ w360]
                  frame False {
                  }
                  frame True {
                    n144 = disable-structure shown="Disabled" {
                      disable-tunnel: w363 -> [w381 _]
                      disable-tunnel: w362 -> [w376 _]
                      disable-tunnel: w361 -> [w374 _]
                      disable-tunnel: w360 -> [w373 _]
                      disable-tunnel: w359 -> [w370 _]
                      disable-tunnel: w358 -> [w369 _]
                      disable-tunnel: [w368 _] -> w357
                      disable-tunnel: w356 -> [w367 _]
                      disable-tunnel: w355 -> [w366 _]
                      disable-tunnel: w354 -> [w365 _]
                      frame Disabled {
                        w364 = TRUE ("x")
                        # "TODO"
                        # "sweep if CH1 = true"
                        n145 = Not Equal?(x=w367, y=w381) -> (x != y?=w379:bool)
                        n146 = while {
                          tunnel: w374 -> [w392]
                          tunnel: w373 -> [w390]
                          tunnel: [w383] -> w372
                          i -> [w391]
                          stop <- w384 stop-if-true
                          # "determine last end frequency"
                          n147 = Subtract(x=w390, y=w391) -> (x-y=w389:i32)
                          n148 = Index Array(array=w392, index=w389) -> (element=w388:T14)
                          n149 = Unbundle By Name(w388) -> ("CH1"=w385:bool, "f1 [Hz] CH1"=w383:dbl, "time[ms]"=w387:dbl)
                          n150 = Not Equal To 0?(x=w387) -> (x != 0?=w386:bool)
                          n151 = And(x=w385, y=w386) -> (x .and. y?=w384:bool)
                        }
                        n152 = And(x=w376, y=w379) -> (x .and. y?=w380:bool)
                        n153 = Not(x=w376) -> (.not. x?=w377:bool)
                        n154 = Not Equal?(x=w367, y=w372) -> (x != y?=w375:bool)
                        n155 = And(x=w377, y=w375) -> (x .and. y?=w378:bool)
                        n156 = Less?(x=w370, y=w367) -> ()  [unwired: 1 out]
                        n157 = Or(x=w380, y=w378) -> (x .or. y?=w382:bool)
                        n158 = And(x=w364, y=w382) -> ()  [unwired: 1 out]
                        n159 = call "FlexDDS-NG_DCP_Sweep.vi"("f1"=w370, "jump before ramp"=w364, "f0"=w367, "sweep time tolerance (us)"=w365, "sweep time (ms)"=w366, "Channels in"=T18."Channel 1", "initial instruction string"=w369) -> ("appended instruction string out"=w368:string)  [unwired: 4 in]
                      }
                      frame Enabled {
                      }
                    }
                  }
                }
                n160 = case shown="False" w352 {
                  tunnel: [w446 w454] -> w349
                  tunnel: w310 -> [_ w453]
                  tunnel: w313 -> [w445 w452]
                  frame False {
                    # "wait on DROVER if one of the channels\nwait 8ns (1h) before waiting on DROVER"
                    n161 = call "FlexDDS-NG_DCP_Wait_Event.vi"("waiting time [ms]"=8e-06, "Channels in"=T18."Both channels", "appended instruction string in"=w445) -> ("appended instruction string"=w447:string)  [unwired: 8 in]
                    n162 = call "FlexDDS-NG_DCP_Wait_Event.vi"("Event 1"=T19."DROVER", "Channels in"=T18."Both channels", "appended instruction string in"=w447) -> ("appended instruction string"=w446:string)  [unwired: 8 in]
                  }
                  frame True {
                    # "do not wait on DROVER only if CH0\nand CH1 are false"
                    n163 = call "FlexDDS-NG_DCP_Wait_Event.vi"("waiting time [ms]"=w453, "appended instruction string in"=w452) -> ("appended instruction string"=w454:string)  [unwired: 9 in]
                  }
                }
              }
            }
          }
        }
      }
      n164 = Concatenate Strings(w208) -> (w206:string)
      n165 = Format Into String(initial string=w205, w206) -> (resulting string=w207:string)  [unwired: 2 in, 1 out]
    }
    frame #4 {
      # "start"
      n166 = call "FlexDDS-NG_DCP_StartStop.vi"("initial instruction string"=w455) -> ("appended instruction string"=w456:string)  [unwired: 10 in]
    }
  }
  n167 = call "FlexDDS-NG_USB_VISA_Open.vi"("FlexDDS-NG USB VISA resource name (COM)"="FlexDDS-NG USB VISA resource name (COM)") -> ("error out"=w3:errorcluster, "FlexDDS-NG USB VISA resource name out"=w5:refnum<visa-resource-name>)  [unwired: 9 in]
  n168 = VISA Write(VISA resource name=w5, write buffer=w22, error in (no error)=w3) -> (VISA resource name out=w6:refnum<visa-resource-name>, return count=→"return count":u32, error out=w2:errorcluster)
  n169 = VISA Read(VISA resource name=w6, byte count=u32 500, error in (no error)=w2) -> (VISA resource name out=w9:refnum<visa-resource-name>, read buffer=→"read buffer":string, error out=→"error out":errorcluster)  [unwired: 1 out]
  n170 = VISA Close(VISA resource name=w9) -> ()  [unwired: 1 in, 1 out]
  "appended instruction string 2" <- w22
